vi "LightHouse Refrigerator Tool.vi"() -> ()   [LabVIEW 2021]
uses:
  Common/LabVIEW GEA2 Toolkit/GEA3/type defs/Data In.ctl
  Common/LabVIEW GEA2 Toolkit/GEA3/type defs/Source_Destination.ctl
  Common/LabVIEW GEA2 Toolkit/GEA3/type defs/ERD Write Data In.ctl
  Common/LabVIEW GEA2 Toolkit/GEA3/type defs/Data Type.ctl
  Common/LabVIEW GEA2 Toolkit/GEA3/type defs/ERD Read Data Out.ctl
  Common/LabVIEW GEA2 Toolkit/GEA3/type defs/ERD Read Data In.ctl
  Dryer Tool (Commercial 2)/JL Dryer Tool Support/type defs/Programming.ctl
  Dryer Tool (Commercial 2)/JL Dryer Tool Support/type defs/Flash_Results.ctl
  Dryer Tool (Commercial 2)/JL Dryer Tool Support/type defs/Select _Graph_JL.ctl
  Common/GEA2 Script/typedefs/Script Info.ctl
  Dryer Tool (Commercial 2)/JL Dryer Tool Support/UTL_JL Scaling Factor Folder/Controls/ENUM_JL Scaling Factor_.ctl
  <vilib>/Platform/fileVersionInfo.llb/FileVersionInformation.ctl
  Dryer Tool (Commercial 2)/JL Dryer Tool Support/type defs/Choose_ERD_List.ctl
  Common/Diagnostics Decode/Type Defs/Diag_FaultTableStatus.ctl
  Common/Diagnostics Decode/Type Defs/Diag_FaultTableEntry.ctl
  Common/Diagnostics Decode/Type Defs/Diag_EntityManifestType.ctl
  Common/Diagnostics Decode/Type Defs/Diag_FaultSeqEntry.ctl
  Automation2/Product Specific/Clothes Care/Justice League/Product Testcode/Diagnostics/TypeDefs/Centauro Diagnostic V3 SnapShot.ctl
  Dryer Tool (Commercial 2)/JL Dryer Tool Support/type defs/JL_Diagnost V3 Cycle History.ctl
  Dryer Tool (Commercial 2)/JL Dryer Tool Support/type defs/ERD_Graph.ctl
  Dryer Tool (Commercial 2)/JL Dryer Tool Support/type defs/ERDList.ctl
  Dryer Tool (Commercial 2)/JL Dryer Tool Support/type defs/ERD_Loop_States_JL.ctl
  Dryer Tool (Commercial 2)/JL Dryer Tool Support/type defs/Version.ctl
  Dryer Tool (Commercial 2)/JL Dryer Tool Support/type defs/BootloaderVersion.ctl
  Common/LabVIEW GEA2 Toolkit/GEA3/type defs/Data Out.ctl
  D:/Common/LabVIEW GEA2 Toolkit/source/GEA3 DLL Source/GeaCommunication.dll
  Common/LabVIEW GEA2 Toolkit/source/GEA3 DLL Source/GeaCommunication.dll
  Common/GExplorer Support/typedefs/GExplorer_Data_Cluster.ctl
  Dryer Tool (Commercial 2)/JL Dryer Tool Support/type defs/ERD_Data_Loop_Control.ctl
  Dryer Tool (Commercial 2)/JL Dryer Tool Support/type defs/Error_Command.ctl
  Dryer Tool (Commercial 2)/JL Dryer Tool Support/type defs/DAQ_States.ctl
  Dryer Tool (Commercial 2)/JL Dryer Tool Support/type defs/Cont_Send_States.ctl
  Refrigerator Tool Support/Controls/All_Bundled_Data_RT.ctl
  Dryer Tool (Commercial 2)/JL Dryer Tool Support/type defs/ERD_Always_Show_JL.ctl
  Dryer Tool (Commercial 2)/JL Dryer Tool Support/type defs/CSV_File_String_Arrays.ctl
  Dryer Tool (Commercial 2)/JL Dryer Tool Support/type defs/Fault Table Array.ctl
  Dryer Tool (Commercial 2)/JL Dryer Tool Support/type defs/Fault_Table_Info.ctl
  Dryer Tool (Commercial 2)/JL Dryer Tool Support/type defs/DAQ_Control_Command.ctl
  Dryer Tool (Commercial 2)/JL Dryer Tool Support/type defs/ERD_Loop_Control_Command.ctl
  Dryer Tool (Commercial 2)/JL Dryer Tool Support/type defs/GEA2_Control_Command.ctl
  <vilib>/DAQmx/read.llb/DAQmx Read (Digital 1D Bool NChan 1Samp 1Line).vi
  <vilib>/DAQmx/write.llb/DAQmx Write (Analog 1D DBL NChan 1Samp).vi
  <vilib>/DAQmx/write.llb/DAQmx Write (Digital 1D Bool NChan 1Samp 1Line).vi
  Common/LabVIEW GEA2 Toolkit/GEA3/advanced/GEA2 Message Received Event Handler.vi
  <vilib>/DAQmx/create/channels.llb/DAQmx Create Channel (DI-Digital Input).vi
  <vilib>/DAQmx/create/channels.llb/DAQmx Create Channel (AO-Voltage-Basic).vi
  <vilib>/DAQmx/create/channels.llb/DAQmx Create Channel (DO-Digital Output).vi
  <vilib>/DAQmx/miscellaneous.llb/DAQmx Fill In Error Info.vi
  Common/LabVIEW GEA2 Toolkit/GEA3/library/GEA2_Toolkit.lvlib
panel:
  in  "Board Index":u8=1 min=1 max=10 step=1
  in  "Pause(mls)":u32=100
  out "Rate":u32=100
  out "State":T1=enum."Read ERDs"
  in  "Data ON":bool=TRUE
  in  "Stop":bool
  in  "UI Launch":bool
  in  "Tab Control":T2(tab)=enum."ERD List"
  out "CSV File Log Path":path=path "D:/QA/Commercial 2/Dryer_Xolo/ProbandoC2_24-11-21_15-05-37.csv"
  out "Version":T3
  in  "Read ERD List":T4[](array[typedef])=[{"ERD Number"=49, "Data Type"=enum."string"}] {"ERD Number" format="%.0x"}
  in  "Read ERD":bool
  in  "Write ERD List":T5[](array[typedef])=[{"ERD Number"=49, "Data Type"=enum."string", "Data"="01"}] {"ERD Number" format="%.0x"}
  in  "Write ERD":bool
  out "Read ERD Data Out":T7[](array[typedef])=[{"ERD Number"=49, "Data"="00 00 00 16"}] {"ERD Number" format="%.0x"}
  out "Boot Loader Version":T8
  in  "GEA Inputs":T9={"Source"=229, "Destination"=2} {"Destination" format="%.0x"; "Source" format="%.0x"}
  in  "Exit Botloader":bool
  in  "Enum":enum16{"All", "MC", "UI"}(ring)
  in  "Entry Botloader":bool
  out "FileVersionInfo":T10
  out "LabView/Version Number":string
  in  "Tool Version":bool=TRUE
  out "GEA2 Log":string
  in  "Save Log":bool
  in  "GEA2 Log Length":i32=100000
  in  "Clear":bool
  in  "Ignore this CMD":string
  in  "Filter Data":bool=TRUE
  in  "Programming":T11={"Program"=FALSE, "File Path"=path "", "Program Ind"=FALSE, "Reset Board"=FALSE, "Enter Bootloader"=FALSE, "Result"=9} {"Result" items=["ImageRejected", "BoardNotFound", "UnableToGetGeaConfiguration", "WriteToFlashNotAllowed", "ImageDownloadedSuccessfully", "ImagePresent", "WriteToFlashFailed", "EraseFailed", "CrcFailed", ""]}
  in  "Flash Latest":bool
  in  "Send Button":bool
  in  "GEA2 Send":T13={"Source"=228, "Destination"=2, "Command"=0, "Message"=""} {"Command" format="%02x"; "Destination" format="%02x"; "Source" format="%02x"}
  in  "Msg Rate (ms)":u32=1000 min=50 step=50
  in  "Start Send":bool
  out "Converted Data Out":T14 {"CRC" format="%04x"; "Length" format="%02x"; "Command" format="%02x"; "Destination" format="%02x"; "Source" format="%02x"}
  in  "ERD Graph Cntrl":cluster{"ERD 3":T15, "ERD 2":T15, "ERD 1":T15}={"ERD 3"={"ERD #"=62250, "Data Type"=enum."uint32_t", "Scaler"=1024}, "ERD 2"={"ERD #"=62250, "Data Type"=enum."uint32_t", "Scaler"=1024}, "ERD 1"={"ERD #"=62250, "Data Type"=enum."uint32_t", "Scaler"=1024}} {"ERD 1"."Scaler" min=1; "ERD 1"."ERD #" format="%.0x"; "ERD 2"."Scaler" min=1; "ERD 2"."ERD #" format="%.0x"; "ERD 3"."Scaler" min=1; "ERD 3"."ERD #" format="%.0x"}
  in  "ERD Graphing ON":bool
  out "ERD Graph  Ind":T16
  in  "Graphing ON":bool
  in  "Select Graph":T17
  out "Outlet Thermistor":u16(graph)
  out "Filtered Moisture":u16(graph)=768
  out "Raw Moisture":u16(graph)=155
  out "All Loads":u16[][](graph)=[[0, 0, 0, 768, 100, 200, 300, 400, 575, 600, 700]]
  out "ERD 1":dbl(graph)
  out "ERD 2":dbl(graph)
  out "Inlet Thermistor":u16(graph)
  out "ERD 3":dbl(graph)
  in  "Get Faults":bool
  in  "Clear Fault Table Buffer":bool
  in  "Clear Fault Seq Buffer":bool
  out "Fault Sequence Entries":T18[](array[typedef])
  out "Fault Seq Status":T19
  out "Fault Table Entries":T20[](array[typedef])
  out "Fault Table Status":T19
  out "Diagnostic Entity Manifest":T21
  out "Major Version":u8
  out "Minor Version":u8
  out "Fault Set?":bool
  in  "Filter by Count":bool=TRUE
  out "Centauro Fault Snapshot":T22
  in  "LED Control":T23
  in  "Normal Temp V":bool=TRUE
  in  "Manual Inlet":dbl format="%#_13g"
  in  "Manual Outlet":dbl format="%#_13g"
  in  "Init/Scale":T24=enum."Scale Voltage"
  in  "Scalling":T25={"Low  "=1531.0, " High"=6859.0, "Actual Low"=1.0, "Actual High"=4.9}
  in  "Desired FilteredMoisture":dbl=2400.0 min=1000.0 max=6300.0 step=5.0
  out "Drum":bool
  out "Centrifugal Switch":bool caption="Cent SW"
  out "Drum Direction":string
  in  "CentSWControl":bool
  in  "CentSWControlType":bool=TRUE
  out "Steam":bool
  out "Drum Light":bool
  out "Outer Coil":bool
  out "Inner/Gas Coil":bool
  in  "Dither (V)":dbl=0.05 min=0.0 max=1.0 step=0.001 format="%_3g"
  in  "Outlet Therm (F)":dbl(knob)=75.0 min=49.0 max=201.0 step=1.0 scale=50.0..200.0
  in  "Inlet Therm (F)":u16(knob)=75 min=49 max=501 step=1 scale=50.0..500.0
  in  "Moisture (V)":dbl(slide)=1.8451000000000002 min=0.0 max=5.0 step=0.0001 scale=0.0..5.0 scale format="%#.2f"
  in  "AC Power":bool=TRUE
  in  "Door Status":bool=TRUE
  in  "Start Signal":bool
  out "DAQ Status":string="Exit"
  in  "Turn On DAQ":bool
  out "DAQ On?":bool
  out "Inlet Voltage":dbl
  out "Outlet Voltage":dbl
  in  "Model":enum16{"Estar Centauro", "GFL"}(ring)
  in  "Get Cycle Data":bool
  in  "Filter by Status Count":bool=TRUE
  out "JL Cycle History":T26
  out "output cluster":T19
  out "Bits":i32
  in  "Script Log Path":path
  in  "Run Script":bool
  out "Script Pass/Fail?":bool
  out "Script Report Text":string
  in  "stop script":bool
  in  "Script Path":path
  out "Script Info":T27 {"Overall Script File Progress" scale=0.0..1.0; "Elapsed time (s)" format="%#.1f"; "Current Script Progress" scale=0.0..1.0}
  out "Script Error Out":errorcluster
  in  "Load ERD List":T28
  in  "ERD Default List":T29=[{"Boolean"=TRUE, "ERD Number"=1792, "ERD Nanme"="Erd_ResetCount", "Data_Type"=enum."string"}] {"ERD Number" format="%x"}
  in  "ERD's List Ticket Testing":T29 {"ERD Number" format="%x"}
  in  "Wifi State":T30(ring)
  in  "Set Wifi State(ERD 6003)":bool
  in  "Turn on Wifi":bool
  in  "Turn off Wifi":bool
  out "Wifi Network State":string
  out "Wifi Password":string
  out "Wifi Network Name":string
  out "Mac Address":string
  in  "Get Wifi Data":bool
  out "Error Out":errorcluster
  in  "Error In":errorcluster
  # "Ver. 0.1"
  # "ERD_Graph_All.ctlERD_Graph_All.ctlMust input av valid ERD# and Data Type DO NOT Leave Blank If no scaler use value of 01"
  # "Filtered Moisture"
  # "Voltage (DAQ)"
  # "Measured Range"
  # "Centrifugal Switch"
  # "On"
  # "Normal"
  # "Off"
  # "Manual"
  # "Wifi State is Writing to ERD 6003 and communicating with the wifi board directly.  It will remain in the state you wrote it to until another command is recieved. \n\nOnly Write to invalid if you are testing the board in Invalid state."
  # "After turning on Wifi , wait about 30 seconds and press the Get Wifi Data button.  Network state should be 1, apmode.\n\nAll this is doing is Writing the ERD 0xF115 Service Request to request connect, or disconnect."
  # "Contact:\n\nTerrance Bradford\nTerrance.Bradford@geappliances.com"
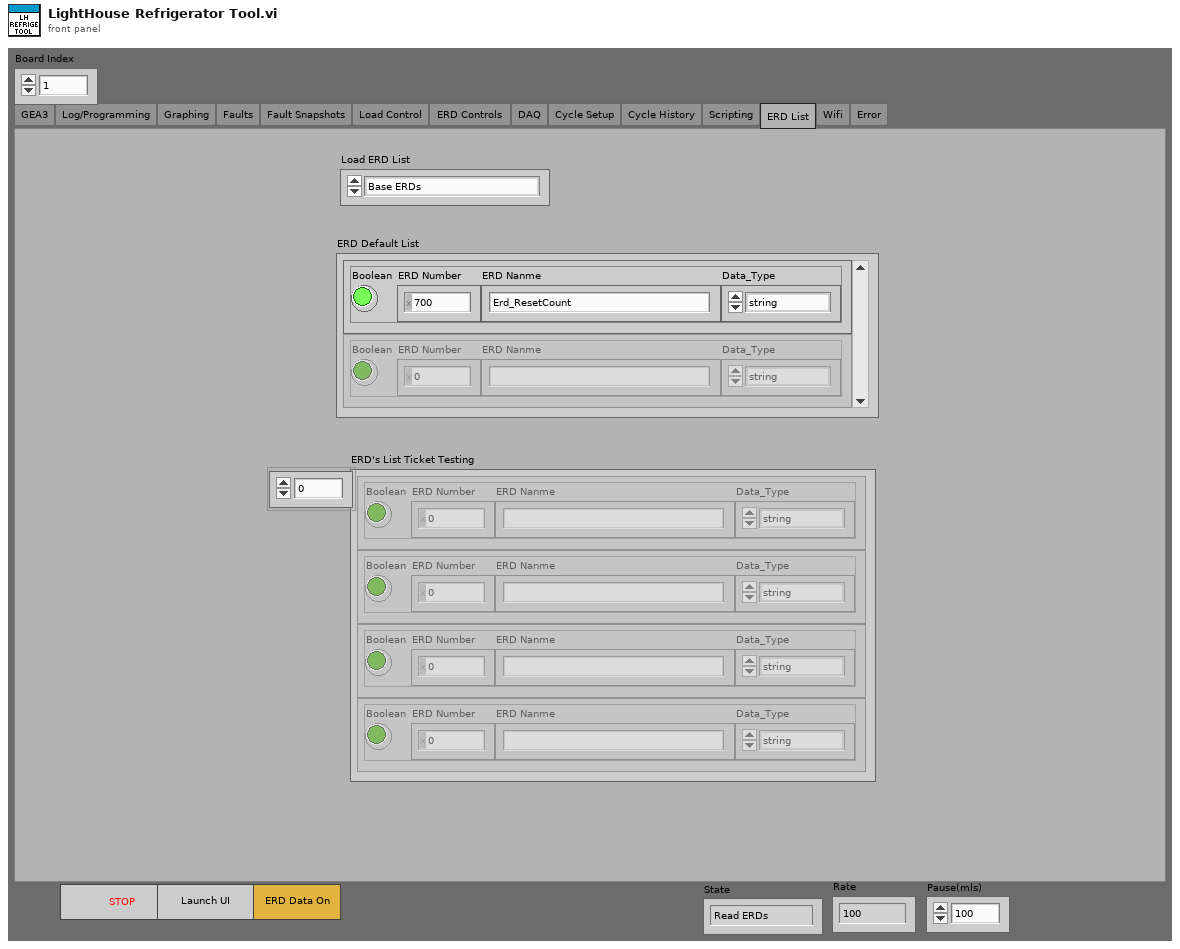
[diagram p1: front panel]
types:
  T1 = typedef "ERD_Loop_States_JL.ctl" = enum16{"Init", "Build ERD Read List", "Read ERDs", "Get Version", "Check Load Size", "Update UI", "Update Graphs", "Read Faults", "Log Data", "Pause", "Shutdown"}
  T2 = enum32{"GEA3", "Log/Programming", "Graphing", "Faults", "Fault Snapshots", "Load Control", "ERD Controls ", "DAQ", "Cycle Setup", "Cycle History", "Scripting", "ERD List", "Wifi", "Error"}
  T3 = typedef "Version.ctl" = cluster{"Build Number":string, "Build Hash ":string, "Application Version":string, "Parametric Version":string, "UI App Version":string}
  T4 = typedef "ERD Read Data In.ctl" = cluster{"ERD Number":u16, "Data Type":enum16{"string", "boolean", "uint8_t", "uint16_t", "uint32_t", "uint64_t", "int8_t", "int16_t", "int32_t", "int64_t"}}
  T5 = typedef "ERD Write Data In.ctl" = cluster{"ERD Number":u16, "Data Type":T6, "Data":string}
  T6 = typedef "Data Type.ctl" = enum16{"string", "boolean", "uint8_t", "uint16_t", "uint32_t", "uint64_t", "int8_t", "int16_t", "int32_t", "int64_t"}
  T7 = typedef "ERD Read Data Out.ctl" = cluster{"ERD Number":u16, "Data":string}
  T8 = typedef "BootloaderVersion.ctl" = cluster{"UI BL Version":string, "MC BL Version":string}
  T9 = typedef "Source_Destination.ctl" = cluster{"Source":u8, "Destination":u8}
  T10 = typedef "FileVersionInformation.ctl" = cluster{"FileVersion":string, "ProductName":string, "InternalName":string, "CompanyName":string, "LegalCopyright":string, "FileDescription":string}
  T11 = typedef "Programming.ctl" = cluster{"Program":bool, "File Path":path, "Program Ind":bool, "Reset Board":bool, "Enter Bootloader":bool, "Result":T12}
  T12 = typedef "Flash_Results.ctl" = i32
  T13 = typedef "Data In.ctl" = cluster{"Source":u8, "Destination":u8, "Command":u8, "Message":string}
  T14 = typedef "Data Out.ctl" = cluster{"Source":u8, "Destination":u8, "Command":u8, "Length":u8, "CRC":u16, "Message":string}
  T15 = typedef "ERD_Graph.ctl" = cluster{"ERD #":u16, "Data Type":T6, "Scaler":u32}
  T16 = cluster{"ERD Value 1":dbl, "ERD Value 2":dbl, "ERD Value 3":dbl}
  T17 = typedef "Select _Graph_JL.ctl" = enum16{"All Loads", "Inlet Thermistor", "Outlet Thermistor", "Raw Moisture", "Filtered Moisture", "ERD 1", "ERD 2", "ERD 3"}
  T18 = typedef "Diag_FaultSeqEntry.ctl" = cluster{"Cycle #":u32, "Time":u32, "F Code":string, "F Active":bool}
  T19 = typedef "Diag_FaultTableStatus.ctl" = cluster{"Cur Index":u16, "Count":u16, "Ov Cnt":u16}
  T20 = typedef "Diag_FaultTableEntry.ctl" = cluster{"Cycle #":u32, "Time":u32, "F Code":string, "F Count":u16, "F Active":bool}
  T21 = typedef "Diag_EntityManifestType.ctl" = cluster{"ID":u8, "Data Ver Maj":u8, "Data Ver Min":u8, "Fault Table?":bool, "Fault Table Snap?":bool, "Fault Seq?":bool, "Fault Seq Snap?":bool, "Cycle History Seq?":bool, "Fault Table Entry Count":u16, "Fault Seq Entry Count":u16, "Cycle History Entry Count":u16, "Cycle Count":u32, "Entity Run Time (Min)":u32}
  T22 = typedef "Centauro Diagnostic V3 SnapShot.ctl" = string[][]
  T23 = cluster{"ALL LEDs ON":bool, "ALL LEDs OFF":bool, "Reset LEDs":bool}
  T24 = typedef "ENUM_JL Scaling Factor_.ctl" = enum16{"Init", "Scale Voltage", "Flush Slope"}
  T25 = cluster{"Low  ":dbl, " High":dbl, "Actual Low":dbl, "Actual High":dbl}
  T26 = typedef "JL_Diagnost V3 Cycle History.ctl" = string[][]
  T27 = typedef "Script Info.ctl" = cluster{"Overall Script File Progress":dbl, "Current Script Progress":dbl, "Script":string, "Test":string, "Elapsed time (s)":dbl, "Done?":bool}
  T28 = typedef "Choose_ERD_List.ctl" = enum16{"Base ERDs", "QA ERDs", "MABE ERD List", "EcoDry Evaluation ERD List", "ClothDampnessCheck ERD List"}
  T29 = typedef "ERDList.ctl" = cluster{"Boolean":bool, "ERD Number":u16, "ERD Nanme":string, "Data_Type":enum16{"string", "boolean", "uint8_t", "uint16_t", "uint32_t", "uint64_t", "int8_t", "int16_t", "int32_t", "int64_t"}}[]
  T30 = enum16{"0 - OFF", "1 - App Mode", "2 - Connecting", "3 - Connected", "4 - Connected Off", "5 - Scanning", "6 - Reconnecting", "255 - Invalid"}
  T31 = typedef "All_Bundled_Data_RT.ctl" = cluster{"Version":T3, "ERD_Always Show":T32, "Personality Set":u8, "CSV File String Arrays":T33, "Fault Table Array ":T34, "Boot Loader Version":T8}
  T32 = typedef "ERD_Always_Show_JL.ctl" = cluster{"Inlet Thermistor":u16, "Machine State":string, "Filtered Moisture":u16, "Cycle Selected":string, "HTR 1 / Inner / Top":bool, "HTR 2 / Outer / Bot":bool, "Door Switch":bool, "Drum Light":bool, "Cycle Engine State":string, "Centrifugal Switch":bool, "Drum Motor":bool, "Cycle Count":u32, "Ext. Tumble":bool, "eDry":bool, "Temp Level":string, "Dryness Level":string, "Time Level":string, "Delay Time (min)":u16, "Steam Refresh":bool, "Damp Alert":bool, "Sub-Cycle":string, "Outlet Thermistor":u16, "Target Moisture":u16, "Remaining Cycle Time":u32, "Raw Moisture":u16, "Cycle Name":string, "My Cycle":bool, "Delay Dry":bool, "Detangle":bool, "Control Lock":bool, "Steam Valve":bool, "Door Latch":bool, "Signal Volume":string, "Tune ID":string, "Restr Detect Status":string, "Vent Restriction":string, "Load Size by Contact":string, "Load Size by Temp":string, "EOC Reason":string, "Sensor Dry Status":string, "Dampness State":string, "Target Voltage Reached":bool, "TrimInhibitR1":bool, "TrimInhibitR2":bool, "TrimBothCoilInhibit":bool, "NormalHeatControl":bool, "HeatControl Request":bool, "Cool Down Status":string, "EcoDryInhibitRelay1":bool, "EcoDryInhibitRelay2":bool, "ReverseDrumInhibitRelay1":bool, "ReverseDrumInhibitRelay2":bool, "OverTempHeaterInhibitRequest":bool, "FallbackHeatControlMethodStatus":bool, "IHC TimeSeconds":u32, "ECT TimeSeconds ":u32, "SC Total Drying Time(S')":u32, "TTR Target Voltage (S')":u32, "TCT Drying Time (S's)":u32, "Drum Motor State":enum16{"Off", "Cw", "Ccw", "Max"}, "Load Size by Ag":string, "MaxFIletered Voltage":u16, "Dry Load Detection":string, "Min Sensing Elapse Sec":u32, "Time Multi Sec X100":u32, "Time Adder  Sec":u32, "Temp Multi EcoDry":string, "Temp Multi ExtraLow":string, "Temp Multi Low ":string, "Temp Multi Medium":string, "Temp Multi High":string, "SmoothMoisture":u16, "Eco Dry SEL Status":string, "Eco Dry SEL Result":string, "Eco Dry Cont Status":string, "Eco Dry Relay1 Timer":string, "Eco Dry Relay2 Timer ":string, "Eco Dry Stage 2 Tans ":u32, "WiFiCommissioningPSt":string, "Payment Method":string}
  T33 = typedef "CSV_File_String_Arrays.ctl" = cluster{"ERD Number Array":string[], "ERD Name Array":string[], "ERD Converted String Data":string[]}
  T34 = typedef "Fault Table Array.ctl" = T35[]
  T35 = typedef "Fault_Table_Info.ctl" = cluster{"Cycle Count":u32, " Runtime (min) ":u32, "Fault Status":string, "Fault ID":string, "Fault Count":u16}
  T36 = typedef "Cont_Send_States.ctl" = enum16{"Run", "Shutdown"}
  T37 = typedef "DAQ_States.ctl" = enum16{"Wait for Init", "Rename Devices", "Verify Hardware", "Initialize", "Run", "Shutdown", "Exit"}
  T38 = typedef "ERD_Data_Loop_Control.ctl" = cluster{"Data":variant, "State":T1}
  T39 = typedef "Error_Command.ctl" = enum16{"Initialize", "Handle Errors", "Report Errors"}
  T40 = typedef "GExplorer_Data_Cluster.ctl" = cluster{"Data":variant, "State":enum16{"Add to Log", "Clear", "Shutdown"}}
  T41 = enum8{"Enabled", "Disabled", "Disabled and Grayed Out"}
  T42 = enum16{"UI Application APL", "UI Parametric APL", "MC APL"}
  T43 = typedef "GEA2_Control_Command.ctl" = enum16{"Initialize", "Shutdown"}
  T44 = typedef "ERD_Loop_Control_Command.ctl" = enum16{"Initialize", "Shutdown"}
  T45 = typedef "DAQ_Control_Command.ctl" = enum16{"Initialize", "Shutdown", "Exit"}
  T46 = enum32{"invalid app kind", "Development System", "Run Time System", "Student Edition", "Embedded LabVIEW", "Evaluation", "Custom"}
  T47 = typedef "eventsource.ctl" = u32
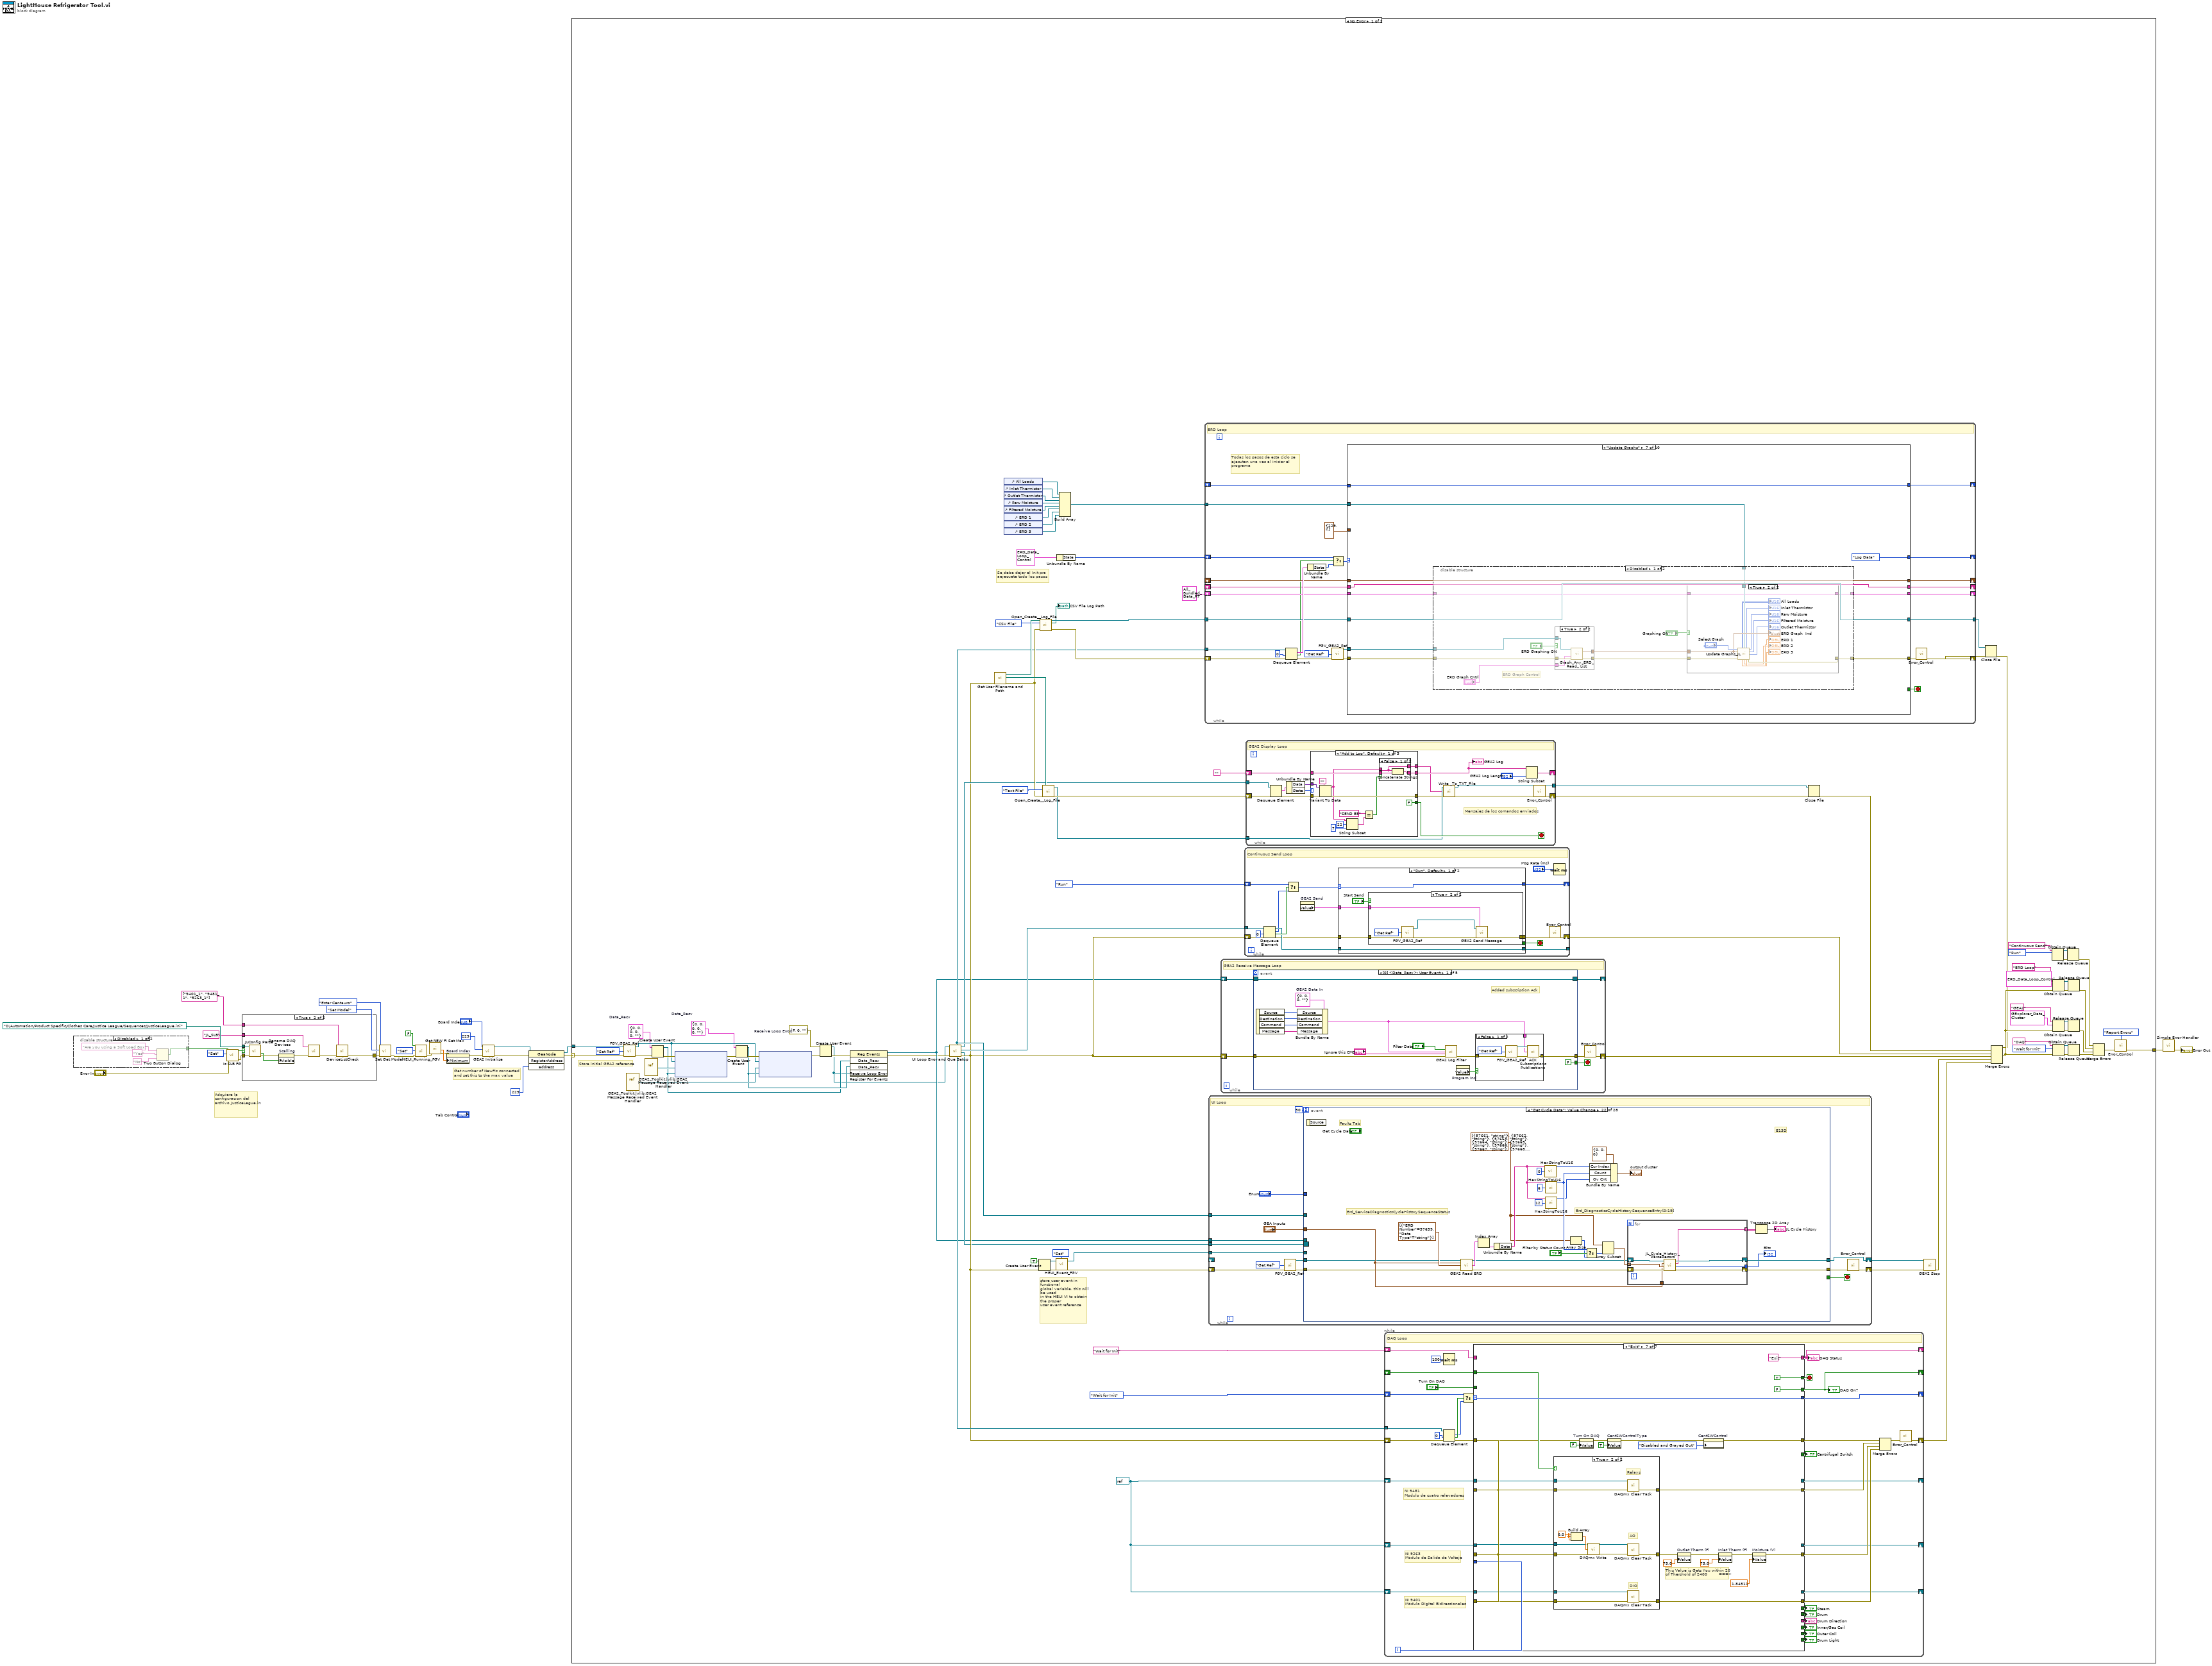
[diagram p0: block diagram]
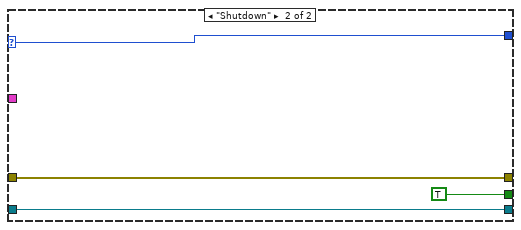
[diagram p5: hidden frame]
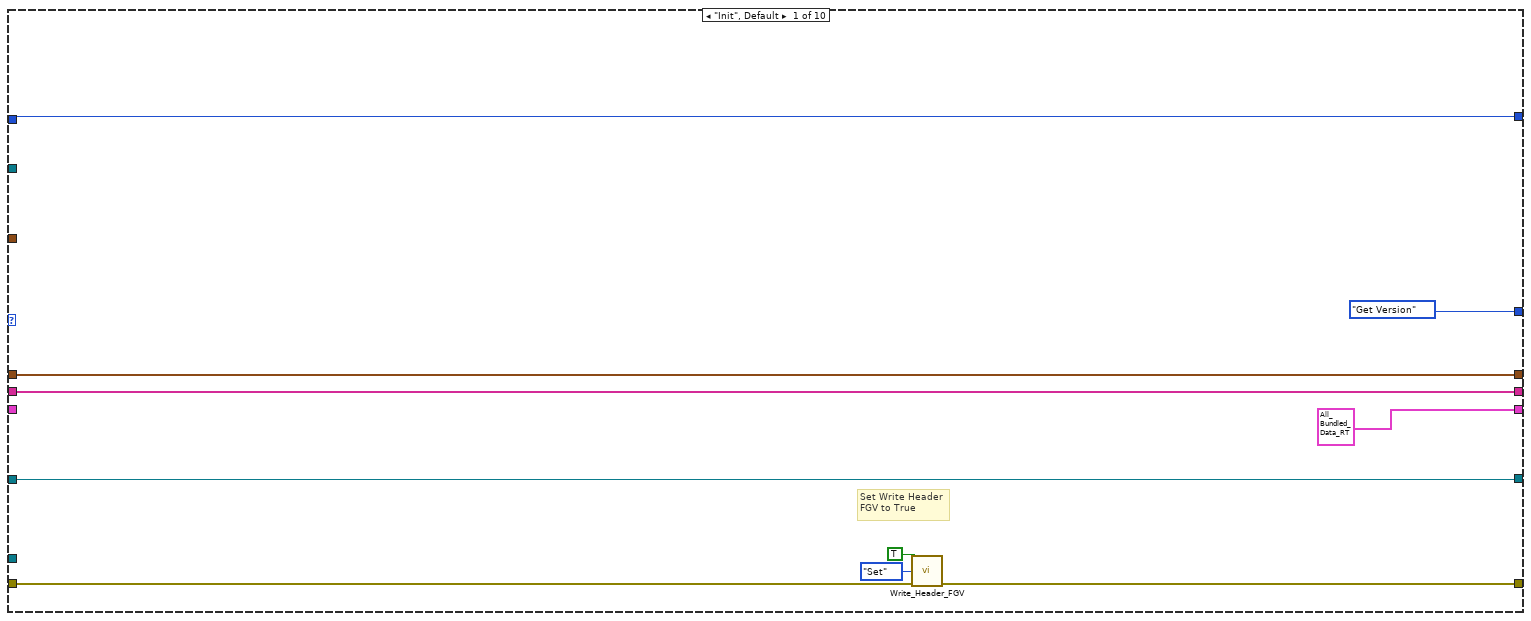
[diagram p6: hidden frame]
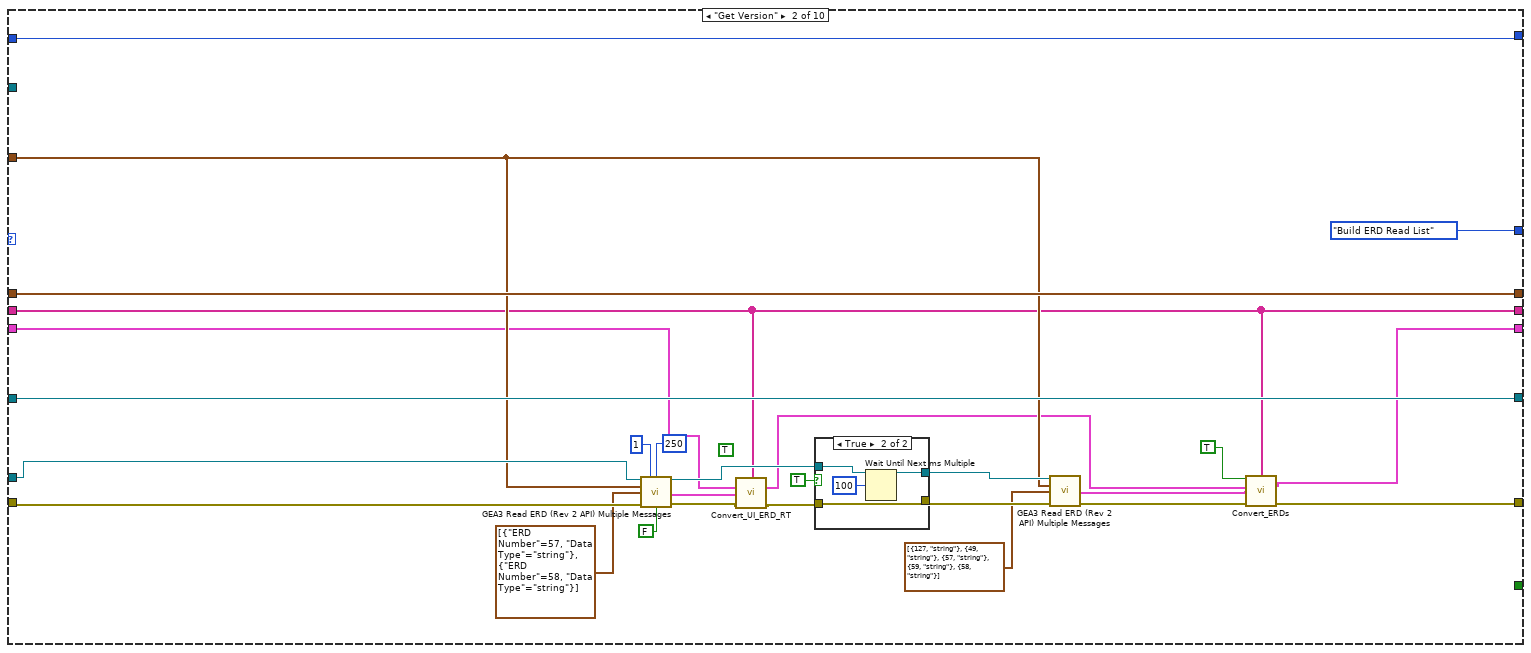
[diagram p7: hidden frame]
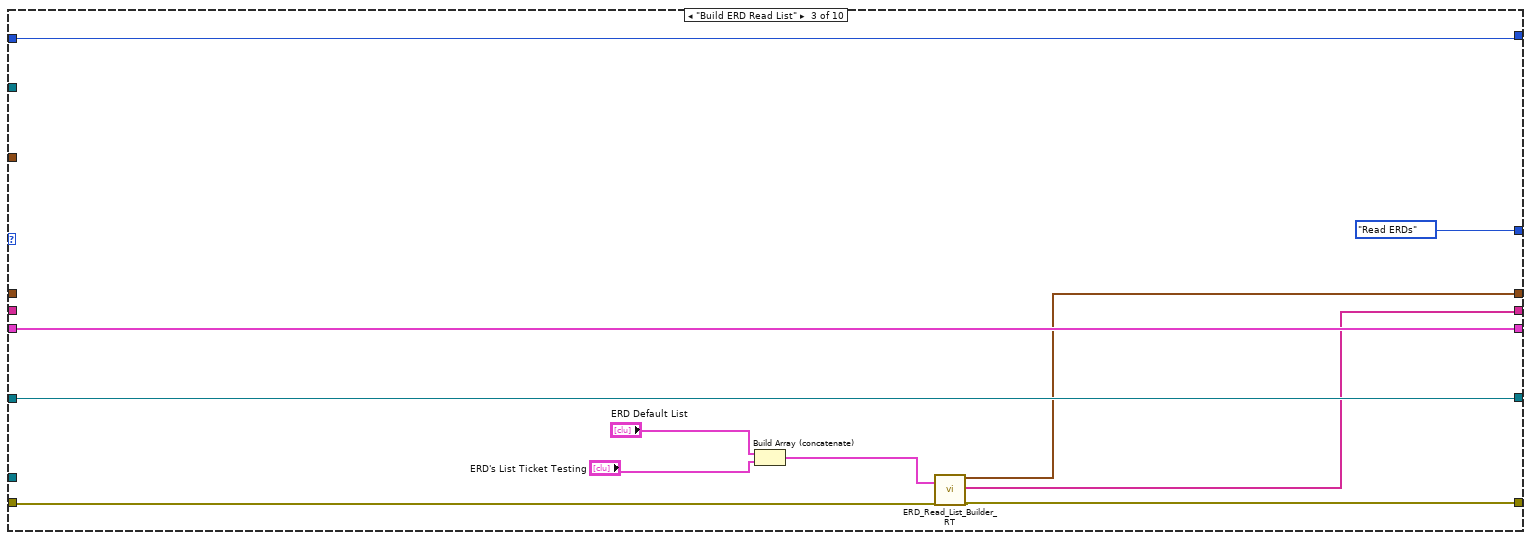
[diagram p9: hidden frame]
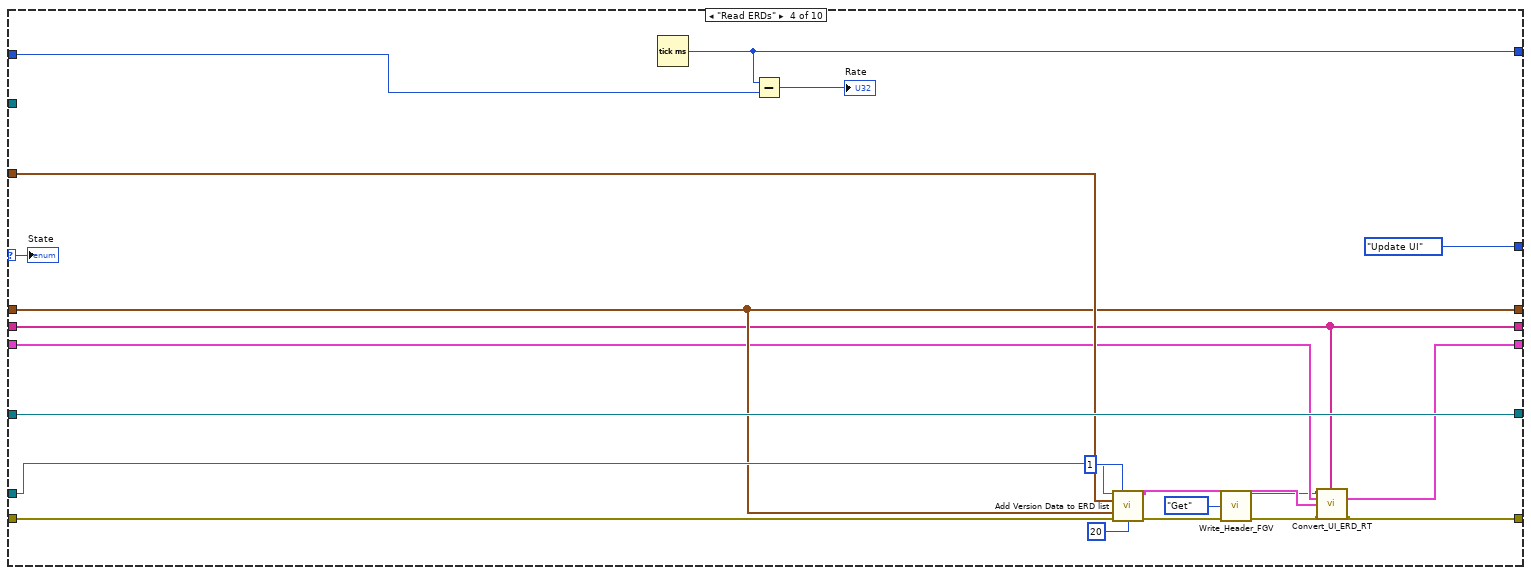
[diagram p10: hidden frame]
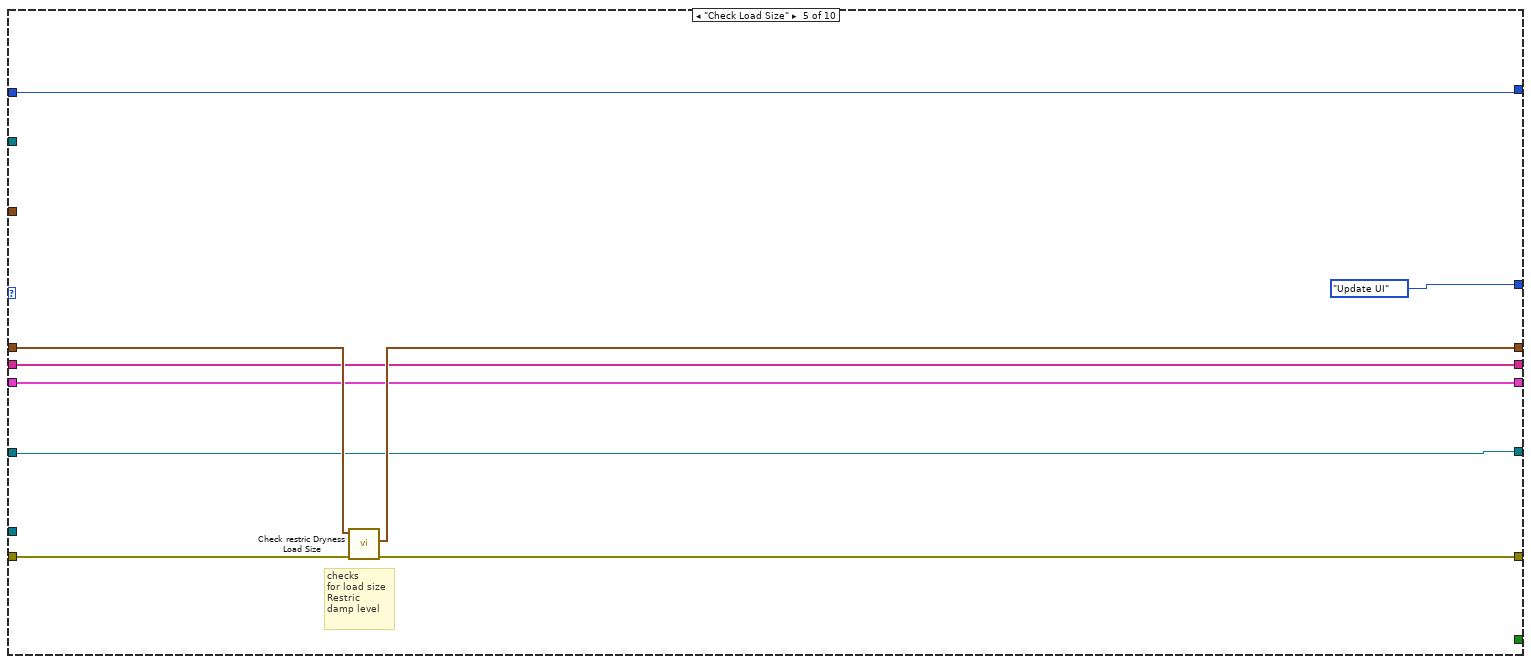
[diagram p11: hidden frame]
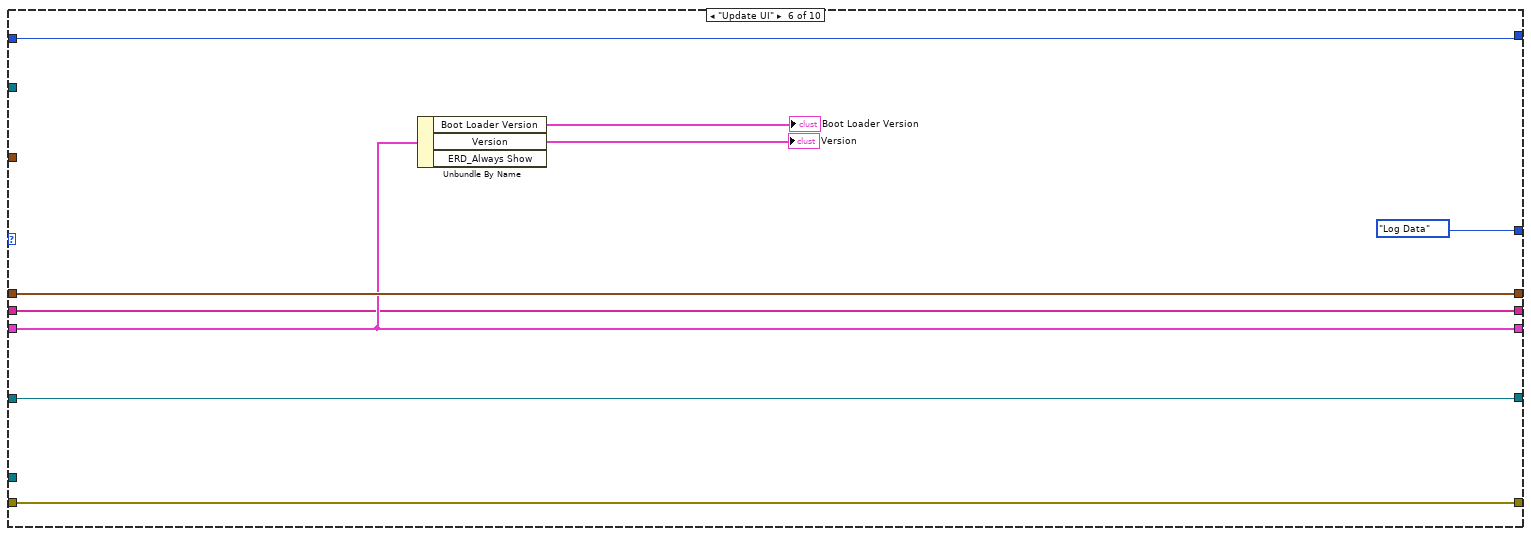
[diagram p12: hidden frame]
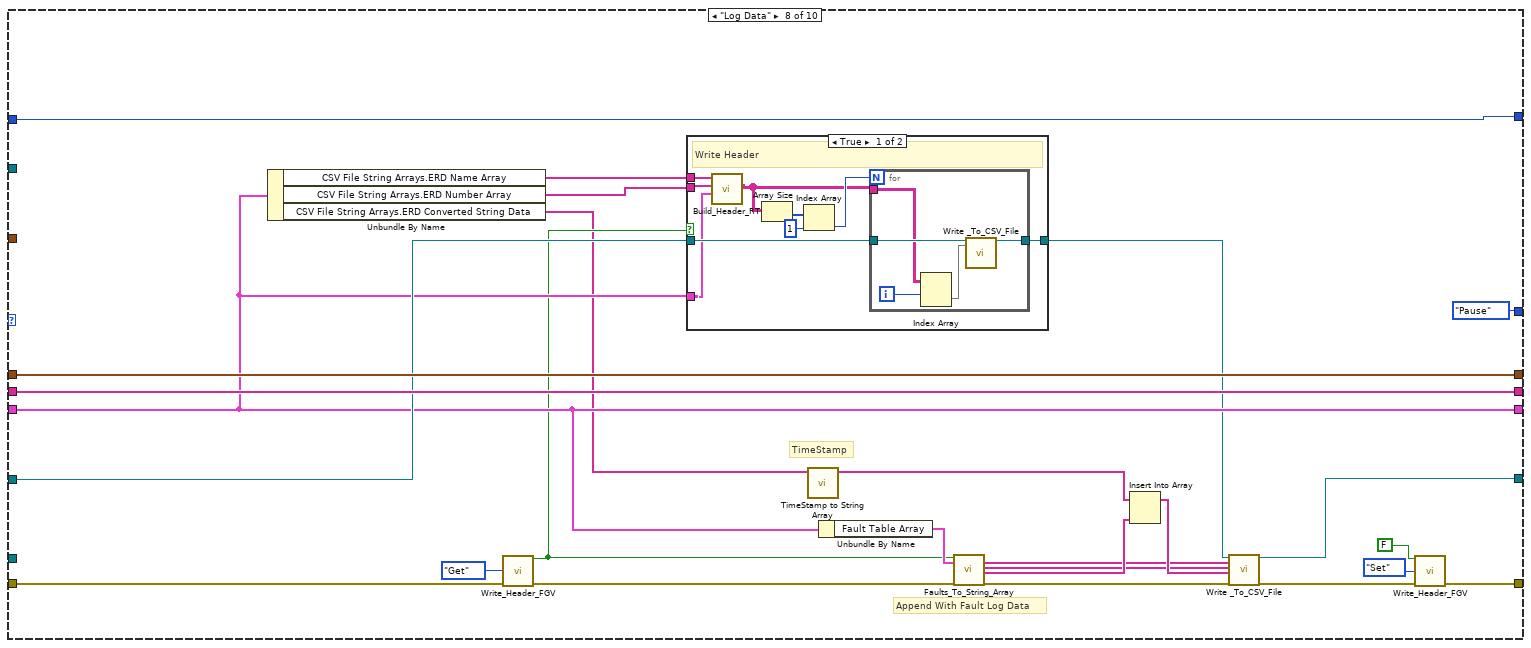
[diagram p16: hidden frame]
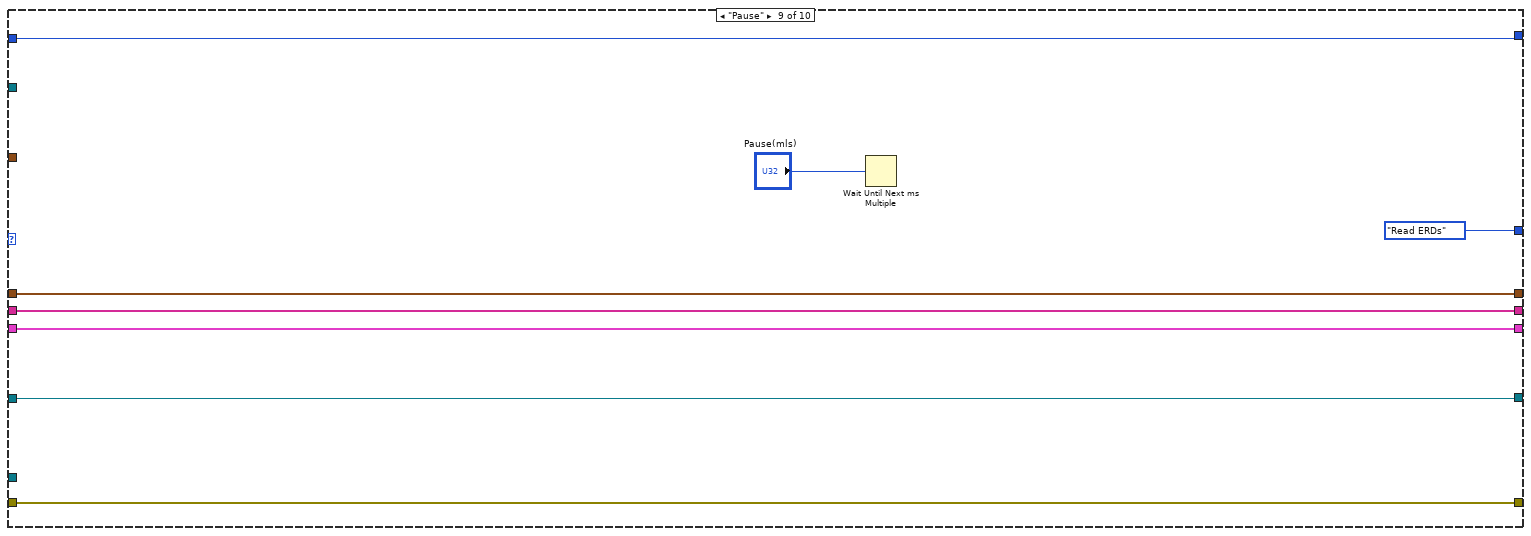
[diagram p18: hidden frame]
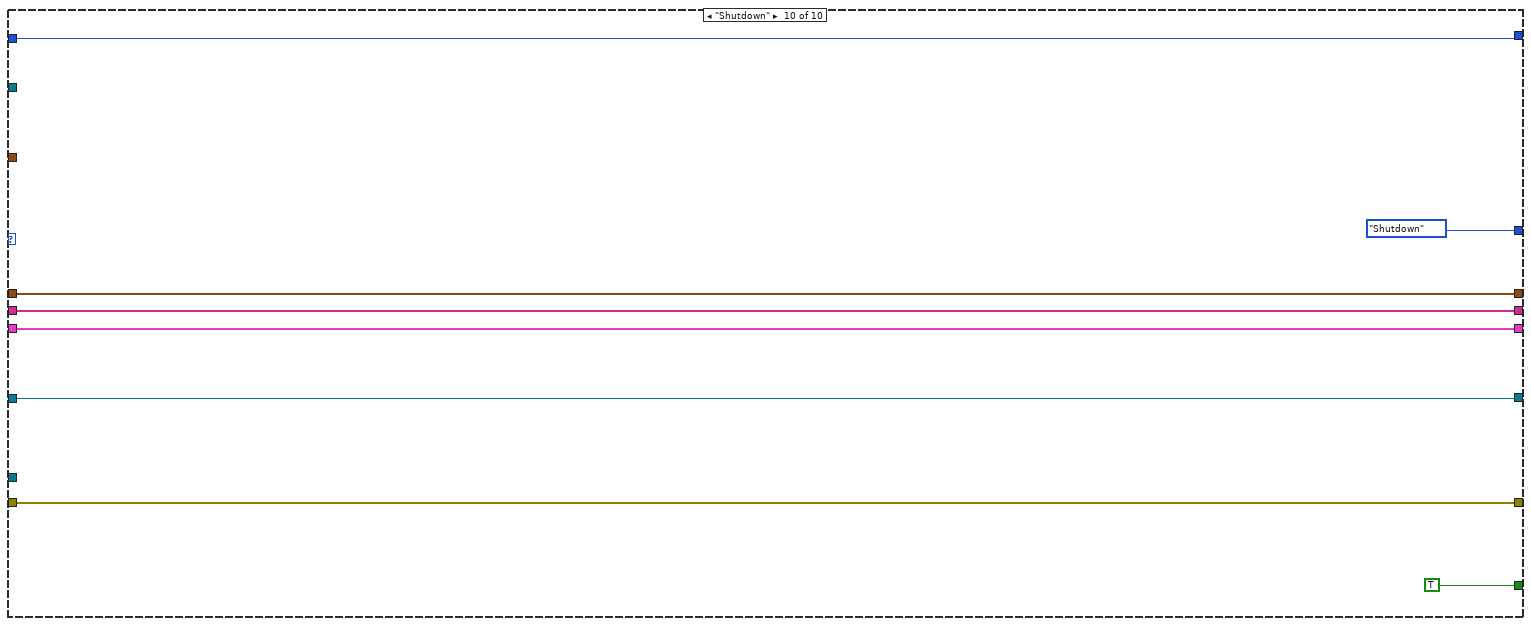
[diagram p19: hidden frame]
diagram:
  # "Adquiere la configuracion del archivo JusticeLegue.in"
  # "Get number of NewFIs connected\nand set this to the max value"
  n1 = disable-structure shown="Disabled" {
    disable-tunnel: [w28 _] -> w16
    frame Disabled {
      n2 = Two Button Dialog(message="Are you using a Soft Load Box?" ("T button name (\"OK\")"), 1:"No" ("F button name (\"Cancel\")"), 2:"Yes" ("message")) -> (T button?=w28:bool)
    }
    frame Enabled {
    }
  }
  n3 = call "Is SLB FG.vi"("Error In"="Error In", "Action"=enum16{"Get", "Set"}."Set", "SLB?"=w16) -> ("Error Out"=w18:errorcluster, "SLB"=w17:bool)  [unwired: 7 in]
  n4 = case shown="True" w17 {
    tunnel: w18 -> [w32 w38]
    tunnel: [w32 w34] -> w13
    tunnel: path "D:/Automation/Product Specific/Clothes Care/Justice League/Sequences/JusticeLeague.ini" ("Config File Path") -> [_ w39]
    tunnel: "JL_SLB" ("cDAQ Name") -> [_ w36]
    tunnel: string[] ["9401_1", "9481_1", "9263_1"] ("Device List") -> [_ w35]
    frame False {
    }
    frame True {
      n5 = call "JLConfig Parse.vi"("Config File Path"=w39, "Error In"=w38) -> ("Calibrate"=w41:bool, "Error Out"=w40:errorcluster)  [unwired: 9 in, 3 out]
      n6 = property on="Scalling" class="Clust (strict)"(error in=w40, "Visible"=w41) -> (error out=w33:errorcluster)  [unwired: 1 in, 1 out]
      n7 = call "Rename DAQ Devices.vi"("cDAQ Name"=w36, "Error In"=w33) -> ("Error Out"=w37:errorcluster)  [unwired: 13 in]
      n8 = call "DeviceListCheck.vi"("Device List"=w35, "Error In"=w37) -> ("Error Out"=w34:errorcluster)  [unwired: 11 in, 2 out]
    }
  }
  n9 = call "Set Get Model.vi"("Error In"=w13, "Action"=enum16{"Set Model", "Get Model"}."Set Model", "Model"=enum16{"Estar Centauro", "GFL"}."Estar Centauro") -> ("Error Out"=w12:errorcluster)  [unwired: 7 in, 1 out]
  n10 = call "HEUI_Running_FGV.vi"("Running?"=FALSE, "Action"=enum16{"Get", "Set"}."Set", "Error In"=w12) -> ("Error Out"=w25:errorcluster)  [unwired: 11 in, 1 out]
  n11 = call "Get NEW FI Set Max.vi"("error in (no error)"=w25) -> ("Error Out"=w8:errorcluster, "Get Max_Out"=w9:dbl)  [unwired: 9 in]
  n12 = property on="Board Index" class="DigNum (strict)"(error in=w8, "Minimum"=w9) -> (error out=w7:errorcluster)  [unwired: 1 in, 1 out]
  n13 = call "GEA2 Initialize.vi"("Board Index"="Board Index", "Source Address"=u8 229, "error in"=w7) -> ("GEA2 Reference Out"=w5:refnum<k24>, "error out"=w2:errorcluster)  [unwired: 10 in, 1 out]
  n14 = invoke class="GeaNode" method="RegisterAddress"(reference=w5, error in=w2, "address"=u8 229 ("Source Address")) -> (reference out=w3:refnum<k24>, error out=w4:errorcluster)  [unwired: 1 in, 2 out]
  n15 = case shown="No Error" w4 {
    selector: w4 -> [w110 w1333]
    tunnel: [w112 w1333] -> w27
    tunnel: w3 -> [w62 _]
    frame No Error {
      w43 = T14 {"Source"=0, "Destination"=0, "Command"=0, "Length"=0, "CRC"=0, "Message"=""}  # Data_Recv
      w45 = T14 {"Source"=0, "Destination"=0, "Command"=0, "Length"=0, "CRC"=0, "Message"=""}  # Data_Recv
      w53 = errorcluster {"status"=FALSE, "code"=0, "source"=""}  # Receive Loop Error
      w67 = refnum<k21> refnum ("task out")
      # "Se debe dejar el Init pra aejecuete todo los pasos"
      # "store user event in functional\nglobal variable, this will be used\nin the HEUI VI to obtain the proper\nuser event reference"
      # "Store initial GEA2 reference"
      n16 = call "FGV_GEA2_Ref.vi"("GEA2 Reference In"=w62, "Action"=enum16{"Set Ref", "Get Ref"}."Set Ref", "Error In"=w110) -> ("GEA2 Reference Out"=w56:refnum<k24>, "Error Out"=w44:errorcluster)  [unwired: 11 in]
      n17 = vi-ref "GEA2_Toolkit.lvlib:GEA2 Message Received Event Handler.vi"() -> (w54:refnum<vi>)
      n18 = vi-ref "GEA2_Toolkit.lvlib:GEA2 Message Received Event Handler.vi"() -> (w55:refnum<vi>)
      n19 = Create User Event(user event datatype=w45, error in=w44) -> (user event=w49:refnum<user-event>, error out=w58:errorcluster)
      n20 = node(w58, w56, w55, w49) -> (w59:errorcluster)  [unwired: 1 in, 1 out]
      n21 = Create User Event(user event datatype=w43, error in=w59) -> (user event=w50:refnum<user-event>, error out=w57:errorcluster)
      n22 = node(w57, w56, w54, w50) -> (w52:errorcluster)  [unwired: 1 in, 1 out]
      n23 = Create User Event(user event datatype=w53, error in=w52) -> (user event=w46:refnum<user-event>, error out=w51:errorcluster)
      n24 = register-events(error in=w51, w49, w50, w46) -> (reference out=w48:refnum<event-registration>, error out=w47:errorcluster)  [unwired: 1 in]
      n25 = call "UI Loop Error and Que Setup.vi"("error in (no error)"=w47, "Receive Loop"=w46) -> ("error out"=w63:errorcluster, "UI Loop Event Registration"=w61:refnum<event-registration>, "Continuous Send Queue"=w83:refnum<queue>, "GEA Display Queue"=w64:refnum<queue>, "Daq Loop queue"=w66:refnum<queue>, "ERD Queue Loop"=w65:refnum<queue>)  [unwired: 4 in]
      n26 = call "Get User Filename and Path.vi"("error in (no error)"=w63) -> ("error out"=w73:errorcluster, "TXT File Path"=w79:path, "CSV File Path"=w81:path)  [unwired: 8 in]
      n27 = control-ref of="All Loads"() -> (w68:refnum<vi>)
      n28 = control-ref of="Inlet Thermistor"() -> (w69:refnum<vi>)
      n29 = control-ref of="Outlet Thermistor"() -> (w70:refnum<vi>)
      n30 = control-ref of="Raw Moisture"() -> (w71:refnum<vi>)
      n31 = control-ref of="Filtered Moisture"() -> (w72:refnum<vi>)
      n32 = control-ref of="ERD 1"() -> (w98:refnum<vi>)
      n33 = control-ref of="ERD 2"() -> (w96:refnum<vi>)
      n34 = control-ref of="ERD 3"() -> (w97:refnum<vi>)
      n35 = Create User Event(user event datatype=TRUE ("Bool"), error in=w63) -> (user event=w105:refnum<user-event>, error out=w106:errorcluster)
      n36 = call "Open_Create__Log_File.vi"("File Path Control"=w81, "Enum"=enum16{"CSV File", "Text File"}."CSV File", "Error In"=w73) -> ("refnum out"=w99:refnum<file>, "File Path"=→"CSV File Log Path":path, "Error Out"=w108:errorcluster)  [unwired: 10 in]
      n37 = call "Open_Create__Log_File.vi"("File Path Control"=w79, "Enum"=enum16{"CSV File", "Text File"}."Text File", "Error In"=w73) -> ("refnum out"=w78:refnum<file>, "Error Out"=w80:errorcluster)  [unwired: 10 in, 1 out]
      n38 = call "HEUI_Event_FGV.vi"("Event In"=w105, "Action"=enum16{"Get", "Set"}."Set", "Error In"=w106) -> ("Event Out"=w102:refnum<user-event>, "Error Out"=w103:errorcluster)  [unwired: 11 in]
      n39 = Unbundle By Name(T38 {"Data"=variant, "State"=enum."Init"} ("Data")) -> ("State"=w100:T1)
      n40 = Build Array(w68, w69, w70, w71, w72, w98, w96, w97) -> (w95:refnum<vi>[])
      n41 = while "Periodic ERD Query Loop" {
        shift-right: [w193] -> w92
        shift-left: w108 -> [w195]
        tunnel: w65 -> [w196]
        shift-right: [w187] -> _
        shift-left: w100 -> [w189]
        shift-right: [w182] -> _
        shift-left: _ -> [w181]
        tunnel: w99 -> [w180]
        tunnel: [w179] -> w90
        shift-right: [w178] -> _
        shift-left: T31 {"Version"={"Build Number"="", "Build Hash "="", "Application Version"="", "Parametric Version"="", "UI App Version"=""}, "ERD_Always Show"={"Inlet Thermistor"=0, "Machine State"="", "Filtered Moisture"=0, "Cycle Selected"="", "HTR 1 / Inner / Top"=FALSE, "HTR 2 / Outer / Bot"=FALSE, "Door Switch"=FALSE, "Drum Light"=FALSE, "Cycle Engine State"="", "Centrifugal Switch"=FALSE, "Drum Motor"=FALSE, "Cycle Count"=0, "Ext. Tumble"=FALSE, "eDry"=FALSE, "Temp Level"="", "Dryness Level"="", "Time Level"="", "Delay Time (min)"=0, "Steam Refresh"=FALSE, "Damp Alert"=FALSE, "Sub-Cycle"="", "Outlet Thermistor"=0, "Target Moisture"=0, "Remaining Cycle Time"=0, "Raw Moisture"=0, "Cycle Name"="", "My Cycle"=FALSE, "Delay Dry"=FALSE, "Detangle"=FALSE, "Control Lock"=FALSE, "Steam Valve"=FALSE, "Door Latch"=FALSE, "Signal Volume"="", "Tune ID"="", "Restr Detect Status"="", "Vent Restriction"="", "Load Size by Contact"="", "Load Size by Temp"="", "EOC Reason"="", "Sensor Dry Status"="", "Dampness State"="", "Target Voltage Reached"=FALSE, "TrimInhibitR1"=FALSE, "TrimInhibitR2"=FALSE, "TrimBothCoilInhibit"=FALSE, "NormalHeatControl"=FALSE, "HeatControl Request"=FALSE, "Cool Down Status"="", "EcoDryInhibitRelay1"=FALSE, "EcoDryInhibitRelay2"=FALSE, "ReverseDrumInhibitRelay1"=FALSE, "ReverseDrumInhibitRelay2"=FALSE, "OverTempHeaterInhibitRequest"=FALSE, "FallbackHeatControlMethodStatus"=FALSE, "IHC TimeSeconds"=0, "ECT TimeSeconds "=0, "SC Total Drying Time(S')"=0, "TTR Target Voltage (S')"=0, "TCT Drying Time (S's)"=0, "Drum Motor State"=enum."Off", "Load Size by Ag"="", "MaxFIletered Voltage"=0, "Dry Load Detection"="", "Min Sensing Elapse Sec"=0, "Time Multi Sec X100"=0, "Time Adder  Sec"=0, "Temp Multi EcoDry"="", "Temp Multi ExtraLow"="", "Temp Multi Low "="", "Temp Multi Medium"="", "Temp Multi High"="", "SmoothMoisture"=0, "Eco Dry SEL Status"="", "Eco Dry SEL Result"="", "Eco Dry Cont Status"="", "Eco Dry Relay1 Timer"="", "Eco Dry Relay2 Timer "="", "Eco Dry Stage 2 Tans "=0, "WiFiCommissioningPSt"="", "Payment Method"=""}, "Personality Set"=0, "CSV File String Arrays"={"ERD Number Array"=[], "ERD Name Array"=[], "ERD Converted String Data"=[]}, "Fault Table Array "=[], "Boot Loader Version"={"UI BL Version"="", "MC BL Version"=""}} ("All_Bundled_Data_Brass") -> [w177]
        tunnel: w95 -> [w176]
        shift-right: [w174] -> _
        shift-left: _ -> [w173]
        shift-right: [w172] -> _
        shift-left: _ -> [w171]
        stop <- w192 stop-if-true
        # "Todas los pasos de esta ciclo se ejecutan una ves al iniciar el programa"
        # "ERD Loop"
        n42 = Dequeue Element(queue=w196, timeout in ms (-1)=0, error in (no error)=w195) -> (element=w184:T38, timed out?=w175:bool, error out=w194:errorcluster)  [unwired: 1 out]
        n43 = Unbundle By Name(w184) -> ("State"=w190:T1)
        n44 = call "FGV_GEA2_Ref.vi"("Action"=enum16{"Set Ref", "Get Ref"}."Get Ref", "Error In"=w194) -> ("GEA2 Reference Out"=w183:refnum<k24>, "Error Out"=w186:errorcluster)  [unwired: 12 in]
        n45 = Select(t=w189, s=w175, f=w190) -> (s? t:f=w188:T1)
        n46 = case shown="\"Update Graphs\"" w188 {
          selector: w188 -> [_ _ _ w268 _ _ _ _ _ _]
          tunnel: w186 -> [w207 w226 w240 w260 w280 w285 w297 w357 w382 w390]
          tunnel: [w201 w217 w241 w252 w278 w285 w296 w356 w382 w390] -> w191
          tunnel: [_ _ _ _ _ _ _ _ _ TRUE] -> w192
          tunnel: T9 {"Source"=229, "Destination"=2} ("ERD Spam GEA Inputs") -> [_ w219 _ w262 _ _ _ _ _ _]
          tunnel: [ERD_Loop_States_JL."Get Version" ("State") ERD_Loop_States_JL."Build ERD Read List" ("State") ERD_Loop_States_JL."Read ERDs" ("State") ERD_Loop_States_JL."Update UI" ("State") ERD_Loop_States_JL."Update UI" ("State") ERD_Loop_States_JL."Log Data" ("State") ERD_Loop_States_JL."Log Data" ("State") ERD_Loop_States_JL."Pause" ("t") ERD_Loop_States_JL."Read ERDs" ("State") ERD_Loop_States_JL."Shutdown" ("State")] -> w187
          tunnel: w183 -> [_ w227 _ w263 _ _ w294 _ _ _]
          tunnel: [w205 w233 w243 w261 w277 w289 w299 w359 w380 w387] -> w182
          tunnel: w181 -> [w205 w233 _ w261 w279 w289 w299 w359 w380 w387]
          tunnel: w180 -> [w204 w232 w249 w270 w276 w286 w298 w353 w379 w386]
          tunnel: [w204 w232 w249 w270 w276 w286 w298 w358 w379 w386] -> w179
          tunnel: [T31 {"Version"={"Build Number"="", "Build Hash "="", "Application Version"="", "Parametric Version"="", "UI App Version"=""}, "ERD_Always Show"={"Inlet Thermistor"=0, "Machine State"="", "Filtered Moisture"=0, "Cycle Selected"="", "HTR 1 / Inner / Top"=FALSE, "HTR 2 / Outer / Bot"=FALSE, "Door Switch"=FALSE, "Drum Light"=FALSE, "Cycle Engine State"="", "Centrifugal Switch"=FALSE, "Drum Motor"=FALSE, "Cycle Count"=0, "Ext. Tumble"=FALSE, "eDry"=FALSE, "Temp Level"="", "Dryness Level"="", "Time Level"="", "Delay Time (min)"=0, "Steam Refresh"=FALSE, "Damp Alert"=FALSE, "Sub-Cycle"="", "Outlet Thermistor"=0, "Target Moisture"=0, "Remaining Cycle Time"=0, "Raw Moisture"=0, "Cycle Name"="", "My Cycle"=FALSE, "Delay Dry"=FALSE, "Detangle"=FALSE, "Control Lock"=FALSE, "Steam Valve"=FALSE, "Door Latch"=FALSE, "Signal Volume"="", "Tune ID"="", "Restr Detect Status"="", "Vent Restriction"="", "Load Size by Contact"="", "Load Size by Temp"="", "EOC Reason"="", "Sensor Dry Status"="", "Dampness State"="", "Target Voltage Reached"=FALSE, "TrimInhibitR1"=FALSE, "TrimInhibitR2"=FALSE, "TrimBothCoilInhibit"=FALSE, "NormalHeatControl"=FALSE, "HeatControl Request"=FALSE, "Cool Down Status"="", "EcoDryInhibitRelay1"=FALSE, "EcoDryInhibitRelay2"=FALSE, "ReverseDrumInhibitRelay1"=FALSE, "ReverseDrumInhibitRelay2"=FALSE, "OverTempHeaterInhibitRequest"=FALSE, "FallbackHeatControlMethodStatus"=FALSE, "IHC TimeSeconds"=0, "ECT TimeSeconds "=0, "SC Total Drying Time(S')"=0, "TTR Target Voltage (S')"=0, "TCT Drying Time (S's)"=0, "Drum Motor State"=enum."Off", "Load Size by Ag"="", "MaxFIletered Voltage"=0, "Dry Load Detection"="", "Min Sensing Elapse Sec"=0, "Time Multi Sec X100"=0, "Time Adder  Sec"=0, "Temp Multi EcoDry"="", "Temp Multi ExtraLow"="", "Temp Multi Low "="", "Temp Multi Medium"="", "Temp Multi High"="", "SmoothMoisture"=0, "Eco Dry SEL Status"="", "Eco Dry SEL Result"="", "Eco Dry Cont Status"="", "Eco Dry Relay1 Timer"="", "Eco Dry Relay2 Timer "="", "Eco Dry Stage 2 Tans "=0, "WiFiCommissioningPSt"="", "Payment Method"=""}, "Personality Set"=0, "CSV File String Arrays"={"ERD Number Array"=[], "ERD Name Array"=[], "ERD Converted String Data"=[]}, "Fault Table Array "=[], "Boot Loader Version"={"UI BL Version"="", "MC BL Version"=""}} ("All_Bundled_Data_Brass") w214 w248 w251 w272 w287 w290 w352 w378 w385] -> w178
          tunnel: w177 -> [_ w211 w248 w255 w272 w287 w293 w352 w378 w385]
          tunnel: w176 -> [_ _ _ _ _ _ w295 _ _ _]
          tunnel: [w200 w210 w242 w253 w274 w284 w292 w355 w377 w384] -> w174
          tunnel: w173 -> [w200 w210 _ w253 w274 w284 w292 w355 w377 w384]
          tunnel: [w199 w231 w247 w267 w273 w283 w291 w354 w376 w383] -> w172
          tunnel: w171 -> [w199 w231 w247 w266 w273 w283 w291 w354 w376 w383]
          frame "Init", Default {
            # "Set Write Header\nFGV to True"
            n47 = call "Write_Header_FGV.vi"("Write Header ? In"=TRUE, "Action"=enum16{"Get", "Set"}."Set", "Error In"=w207) -> ("Error Out"=w201:errorcluster)  [unwired: 11 in, 1 out]
          }
          frame "Get Version" {
            (unwired) TRUE ("New Header?")
            n48 = call "GEA3 Read ERD (Rev 2 API) Multiple Messages.vi"("GEA2 Reference In"=w227, "Retry Count"=1 ("# of Iterations (Should be 2 except JL)"), "Read Timeout (ms)"=u32 250, "GEA Inputs"=w219, "Read ERD List"=T4[] [{"ERD Number"=57, "Data Type"=enum."string"}, {"ERD Number"=58, "Data Type"=enum."string"}] ("Read ERD List MC"), "Error In"=w226, "Verify ERD Response?"=FALSE) -> ("GEA2 Reference Out"=w225:refnum<k24>, "ERD Data Out"=w212:cluster{"ERD Number":u16, "Data":string}[], "Error Out"=w213:errorcluster)  [unwired: 5 in, 1 out]
            n49 = call "Convert_UI_ERD_RT.vi"("ERD Name"=w210, "All_Bundled_Data_Brass"=w211, "Array"=w212, "Error In"=w213) -> ("All_ERD_Data_Bundled_Brass"=w208:T31, "Error Out"=w209:errorcluster)  [unwired: 10 in]
            n50 = case shown="True" TRUE {
              tunnel: [w235 w239] -> w223
              tunnel: w209 -> [w235 w239]
              tunnel: [w236 w238] -> w222
              tunnel: w225 -> [w236 w238]
              frame False {
              }
              frame True {
                n51 = Wait Until Next ms Multiple(millisecond multiple=u32 100) -> ()  [unwired: 1 out]
              }
            }
            n52 = call "GEA3 Read ERD (Rev 2 API) Multiple Messages.vi"("GEA2 Reference In"=w222, "GEA Inputs"=w219, "Read ERD List"=T4[] [{"ERD Number"=127, "Data Type"=enum."string"}, {"ERD Number"=49, "Data Type"=enum."string"}, {"ERD Number"=57, "Data Type"=enum."string"}, {"ERD Number"=59, "Data Type"=enum."string"}, {"ERD Number"=58, "Data Type"=enum."string"}] ("Read ERD List MC"), "Error In"=w223) -> ("ERD Data Out"=w216:cluster{"ERD Number":u16, "Data":string}[], "Error Out"=w218:errorcluster)  [unwired: 8 in, 2 out]
            n53 = call "Convert_ERDs.vi"("New Header?"=TRUE, "ERD Name"=w210, "All_Bundled_Data_Brass"=w208, "Array"=w216, "Error In"=w218) -> ("All_ERD_Data_Bundled_Brass"=w214:T31, "Error Out"=w217:errorcluster)  [unwired: 9 in]
          }
          frame "Build ERD Read List" {
            n54 = Build Array (concatenate)("ERD Default List", "ERD's List Ticket Testing") -> (w244:T29)
            n55 = call "ERD_Read_List_Builder_RT.vi"("ERD Read List ALL"=w244, "Error In"=w240) -> ("Read ERD List"=w243:T4[], "ERD Name"=w242:string[], "Error Out"=w241:errorcluster)  [unwired: 15 in]
          }
          frame "Read ERDs" {
            n56 = Tick Count (ms)() -> (millisecond timer value=w267:u32)
            n57 = Subtract(x=w267, y=w266) -> (x-y=→"Rate":u32)
            n58 = call "Add Version Data to ERD list.vi"(".NET Refnum in"=w263, "# of Iterations (Should be 2 except JL)"=1, "GEA Inputs"=w262, "Read ERD List MC"=w261, "error in (no error)"=w260, "#ERDs per message"=20) -> ("ERD Data Out out"=w256:T7[], "error out"=w259:errorcluster)  [unwired: 8 in]
            n59 = call "Write_Header_FGV.vi"("Action"=enum16{"Get", "Set"}."Get", "Error In"=w259) -> ("Write Header ? Out"=w254:bool, "Error Out"=w257:errorcluster)  [unwired: 12 in]
            n60 = call "Convert_UI_ERD_RT.vi"("New Header?"=w254, "ERD Name"=w253, "All_Bundled_Data_Brass"=w255, "Array"=w256, "Error In"=w257) -> ("All_ERD_Data_Bundled_Brass"=w251:T31, "Error Out"=w252:errorcluster)  [unwired: 9 in]
            "State" <- w268
          }
          frame "Check Load Size" {
            # "checks \nfor load size \nRestric\ndamp level"
            n61 = call "Check restric Dryness Load Size.vi"("Error In"=w280, "Read ERD List"=w279) -> ("Error Out"=w278:errorcluster, "New ERD Data"=w277:T4[])  [unwired: 8 in]
          }
          frame "Update UI" {
            n62 = Unbundle By Name(w287) -> ("Boot Loader Version"=→"Boot Loader Version":T8, "Version"=→"Version":T3)  [unwired: 1 out]
          }
          frame "Update Graphs" {
            n63 = disable-structure shown="Disabled" {
              disable-tunnel: w297 -> [w311 _]
              disable-tunnel: [w309 _] -> w296
              disable-tunnel: w295 -> [w306 _]
              disable-tunnel: w294 -> [w305 _]
              disable-tunnel: w293 -> [w304 _]
              disable-tunnel: [w303 _] -> w290
              frame Disabled {
                # "ERD Graph Control"
                n64 = case shown="True" "ERD Graphing ON" {
                  tunnel: w311 -> [w328 w333]
                  tunnel: [w328 w332] -> w310
                  tunnel: "ERD Graph Cntrl" -> [_ w331]
                  tunnel: [_ w330] -> w307
                  tunnel: w305 -> [_ w329]
                  frame False {
                  }
                  frame True {
                    n65 = call "Graph_Any_ERD_ Read_ List.vi"("GEA2 Reference In"=w329, "ERD Graph Cntrl"=w331, "Error In"=w333) -> ("ERD Graph  Ind"=w330:T16, "Error Out"=w332:errorcluster)  [unwired: 10 in, 1 out]
                  }
                }
                n66 = case shown="True" "Graphing ON" {
                  tunnel: w310 -> [w312 w327]
                  tunnel: [w312 w326] -> w309
                  tunnel: w307 -> [_ w324]
                  tunnel: w306 -> [_ w323]
                  tunnel: w304 -> [w313 w319]
                  tunnel: [w313 w319] -> w303
                  frame False {
                  }
                  frame True {
                    n67 = call "Update Graphs_JL.vi"("Select Graph"="Select Graph", "appended array"=w323, "ERD Graph  Ind 2"=w324, "Error In"=w327) -> ("All Loads"=→"All Loads":u16[][], "Inlet Thermistor"=→"Inlet Thermistor":u16, "Raw Moisture"=→"Raw Moisture":u16, "Filtered Moisture"=→"Filtered Moisture":u16, "Outlet Thermistor"=→"Outlet Thermistor":u16, "ERD 3"=→"ERD 3":dbl, "ERD 2"=→"ERD 2":dbl, "ERD 1"=→"ERD 1":dbl, "Error Out"=w326:errorcluster)  [unwired: 3 in]
                    "ERD Graph  Ind" <- w324
                  }
                }
              }
              frame Enabled {
              }
            }
          }
          frame "Log Data" {
            # "TimeStamp"
            # "Append With Fault Log Data"
            n68 = Unbundle By Name(w352) -> ("CSV File String Arrays.ERD Name Array"=w350:string[], "CSV File String Arrays.ERD Number Array"=w334:string[], "CSV File String Arrays.ERD Converted String Data"=w339:string[])
            n69 = call "Write_Header_FGV.vi"("Action"=enum16{"Get", "Set"}."Get", "Error In"=w357) -> ("Write Header ? Out"=w340:bool, "Error Out"=w345:errorcluster)  [unwired: 12 in]
            n70 = case shown="True" w340 {
              tunnel: w350 -> [w362 _]
              tunnel: w353 -> [w368 w374]
              tunnel: [w367 w374] -> w338
              tunnel: w352 -> [w363 _]
              tunnel: w334 -> [w361 _]
              frame True {
                # "Write Header"
                n71 = call "Build_Header_RT.vi"("All_Bundled_Data_Brass"=w363, "ERD Number Array In"=w361, "ERD Name Array In"=w362) -> ("ERD Name Array out 2"=w360:string[][])  [unwired: 8 in]
                n72 = Array Size(array=w360) -> (size(s)=w366:i32[])
                n73 = Index Array(array=w366, index=1) -> (element=w364:i32)
                n74 = for {
                  N: w364 -> [_]
                  tunnel: w368 -> [w373]
                  tunnel: [w372] -> w367
                  tunnel: w360 -> [w371]
                  i -> [w370]
                  n75 = Index Array(array=w371, index (row)=w370) -> (element=w369:string[])  [unwired: 1 in]
                  n76 = call "Write _To_CSV_File.vi"("Refnum In"=w373, "ERD Name"=w369) -> ("Refnum Out"=w372:refnum<file>)  [unwired: 15 in, 2 out]
                }
              }
              frame False {
              }
            }
            n77 = call "TimeStamp to String Array.vi"("String Array In"=w339) -> ("String Array Out"=w337:string[])  [unwired: 10 in]
            n78 = Unbundle By Name(w352) -> ("Fault Table Array"=w341:T34)
            n79 = call "Faults_To_String_Array.vi"("Write Header ?"=w340, "Fault Table Entry"=w341, "Error In"=w345) -> ("Fault Header String Array"=w336:string[], "Fault ERD Number String Array"=w335:string[], "Fault Data String Array"=w344:string[], "Error Out"=w342:errorcluster)  [unwired: 13 in]
            n80 = Insert Into Array(array=w337, new element=w344) -> (w343:string[])  [unwired: 1 in]
            n81 = call "Write _To_CSV_File.vi"("Refnum In"=w338, "ERD Name"=w336, "ERD Number"=w335, "ERD Data"=w343, "Error In"=w342) -> ("Refnum Out"=w358:refnum<file>, "Error Out"=w347:errorcluster)  [unwired: 12 in, 1 out]
            n82 = call "Write_Header_FGV.vi"("Write Header ? In"=FALSE, "Action"=enum16{"Get", "Set"}."Set", "Error In"=w347) -> ("Error Out"=w356:errorcluster)  [unwired: 11 in, 1 out]
          }
          frame "Pause" {
            n83 = Wait Until Next ms Multiple(millisecond multiple="Pause(mls)") -> ()  [unwired: 1 out]
          }
          frame "Shutdown" {
          }
        }
        n84 = call "Error_Control.vi"("Error In"=w191) -> ("Error Out"=w193:errorcluster)  [unwired: 14 in]
      }
      n85 = while "UI Loop" {
        shift-right: [w685] -> w135
        shift-left: w103 -> [w679]
        shift-right: [w687] -> w134
        shift-left: _ -> [_]
        tunnel: w61 -> [w686]
        tunnel: w102 -> [w676]
        tunnel: w65 -> [w675]
        tunnel: w48 -> [w674]
        stop <- w684 stop-if-true
        # "UI Loop"
        n86 = call "FGV_GEA2_Ref.vi"("Action"=enum16{"Set Ref", "Get Ref"}."Get Ref", "Error In"=w679) -> ("GEA2 Reference Out"=w678:refnum<k24>, "Error Out"=w680:errorcluster)  [unwired: 12 in]
        n87 = event shown="[21] \"Get Cycle Data\": Value Change" {
          selector: w686 -> [_ _ _ _ _ _ _ _ _ _ _ _ _ _ _ _ _ _ _ _ _ _ _ _ _ _ _ _]
          dyn-events: _ -> [_ _ _ _ _ _ _ _ _ _ _ _ _ _ _ _ _ _ _ _ _ _ _ _ _ _ _ _]
          timeout: 50 -> [_ _ _ _ _ _ _ _ _ _ _ _ _ _ _ _ _ _ _ _ _ _ _ _ _ _ _ _]
          tunnel: [w690 w698 w712 w733 w734 w738 w745 w760 w778 w821 w874 w880 w892 w902 _ w917 w961 w1041 w1048 w1063 w1095 w1112 w1141 w1151 w1164 w1175 _ w1232] -> w683
          tunnel: w680 -> [w691 w700 w715 w730 w734 w739 w744 w759 w786 w826 w879 w890 w896 w903 w908 w914 w963 w1039 w1049 w1064 w1096 w1109 w1142 w1159 w1164 w1182 w1188 w1234]
          tunnel: [_ _ _ _ _ _ _ _ _ _ _ _ _ _ _ _ _ _ _ _ _ _ _ TRUE _ _ _ _] -> w684
          tunnel: w678 -> [w692 w701 w714 w732 w735 w742 w748 _ w787 w827 w878 w889 _ w901 _ w926 w964 _ w1046 w1061 w1099 w1110 _ w1162 w1165 w1181 w1189 w1233]
          tunnel: [w693 w699 w713 w732 w735 w743 w749 _ _ _ _ w888 _ w901 _ _ w960 _ w1047 w1062 w1097 w1111 _ w1162 w1165 w1176 _ w1231] -> w687
          tunnel: "GEA Inputs" -> [_ _ _ _ _ w741 w747 _ _ _ _ _ _ _ _ _ w965 _ w1045 w1065 w1098 w1113 _ _ _ _ w1190 _]
          tunnel: w676 -> [_ _ _ _ _ _ _ _ w783 w825 _ _ _ _ _ w911 _ _ _ _ _ _ _ _ _ _ _ _]
          tunnel: w675 -> [_ _ _ _ _ _ _ _ w777 w822 w873 _ _ _ _ w912 _ w1037 _ _ _ _ w1139 _ _ _ _ _]
          tunnel: w674 -> [_ _ _ _ _ _ _ _ _ _ _ _ _ _ _ _ _ _ _ _ _ _ _ _ _ _ _ _]
          tunnel: "Enum" -> [_ w694 w711 _ _ _ _ _ _ _ _ _ _ _ _ _ _ _ _ _ _ _ _ _ _ _ _ _]
          event "Send Button": Value Change {
            # "GEA2 Tab"
            n88 = event-data() -> ()  [unwired: 1 in, 1 out]
            n89 = call "GEA2 Send and Receive Message.vi"("GEA2 Reference In"=w692, "Input Data"="GEA2 Send", "Error In"=w691) -> ("GEA2 Reference Out"=w693:refnum<k24>, "Converted Data Out"=→"Converted Data Out":T14, "Error Out"=w690:errorcluster)  [unwired: 9 in, 1 out]
          }
          event "Entry Botloader": Value Change {
            n90 = event-data() -> ()  [unwired: 1 in, 1 out]
            n91 = case shown="\"All\", Default" w694 {
              tunnel: T13 {"Source"=229, "Destination"=2, "Command"=221, "Message"="07"} ("GEA2 Send") -> [w703 w707 w708]
              tunnel: [w702 w705 w709] -> w695
              frame "All", Default {
                n92 = Bundle By Name(cluster=w703, "Destination"=u8 255) -> (w702:T13)
              }
              frame "MC" {
                n93 = Bundle By Name(cluster=w707, "Destination"=u8 192) -> (w705:T13)
              }
              frame "UI" {
                n94 = Bundle By Name(cluster=w708, "Destination"=u8 37) -> (w709:T13)
              }
            }
            n95 = call "GEA2 Send and Receive Message.vi"("GEA2 Reference In"=w701, "Input Data"=w695, "Error In"=w700) -> ("GEA2 Reference Out"=w699:refnum<k24>, "Converted Data Out"=w697:T14, "Error Out"=w698:errorcluster)  [unwired: 9 in, 1 out]
            n96 = Unbundle By Name(w697) -> ()  [unwired: 1 out]
          }
          event "Exit Botloader": Value Change {
            n97 = event-data() -> ()  [unwired: 1 in, 1 out]
            n98 = case shown="\"MC\"" w711 {
              tunnel: T13 {"Source"=229, "Destination"=2, "Command"=221, "Message"="F4 01"} ("GEA2 Send") -> [w719 w723 w724]
              tunnel: [w718 w721 w725] -> w716
              frame "All", Default {
                n99 = Bundle By Name(cluster=w719, "Destination"=u8 255) -> (w718:T13)
              }
              frame "MC" {
                n100 = Bundle By Name(cluster=w723, "Destination"=u8 192) -> (w721:T13)
              }
              frame "UI" {
                n101 = Bundle By Name(cluster=w724, "Destination"=u8 37) -> (w725:T13)
              }
            }
            n102 = call "GEA2 Send and Receive Message.vi"("GEA2 Reference In"=w714, "Input Data"=w716, "Error In"=w715) -> ("GEA2 Reference Out"=w713:refnum<k24>, "Error Out"=w712:errorcluster)  [unwired: 9 in, 2 out]
          }
          event "Clear": Value Change {
            w727 = T40 {"Data"=variant, "State"=enum."Clear"} ("element")
            # "GEA2 Tab"
            n103 = event-data() -> ()  [unwired: 1 in, 6 out]
            n104 = Obtain Queue(name (unnamed)="GEA2", element data type=w727, error in (no error)=w730) -> (queue out=w728:refnum<queue>, error out=w731:errorcluster)  [unwired: 2 in, 1 out]
            n105 = Enqueue Element(queue=w728, element=w727, error in (no error)=w731) -> (error out=w733:errorcluster)  [unwired: 1 in, 2 out]
          }
          event Timeout {
            # "Must have timeout case to give GEA2 FGV a chance to update\nthe GEA2 reference. Otherwise, when we receive an event it may\nbe using a reference that is no longer valid."
            n106 = event-data() -> ()  [unwired: 1 in, 3 out]
          }
          event "Write ERD": Value Change {
            # "Read/Write ERDs Tab"
            n107 = event-data() -> ()  [unwired: 1 in, 1 out]
            n108 = call "GEA3 Write ERD (Rev 2 API) Multiple Messages.vi"("GEA2 Reference In"=w742, "# of Tries"=2 ("Retry Count"), "GEA Inputs"=w741, "Write ERD List"="Write ERD List", "Error In"=w739, "Verify ERD Response?"=TRUE) -> ("GEA2 Reference Out"=w743:refnum<k24>, "Error Out"=w738:errorcluster)  [unwired: 7 in, 1 out]
          }
          event "Read ERD": Value Change {
            # "Read/Write ERDs tab"
            n109 = event-data() -> ()  [unwired: 1 in, 6 out]
            n110 = call "GEA3 Read ERD (Rev 2 API) Multiple Messages.vi"("GEA2 Reference In"=w748, "Retry Count"=2, "GEA Inputs"=w747, "Read ERD List"="Read ERD List", "Error In"=w744, "Verify ERD Response?"=TRUE) -> ("GEA2 Reference Out"=w749:refnum<k24>, "ERD Data Out"=→"Read ERD Data Out":cluster{"ERD Number":u16, "Data":string}[], "Error Out"=w745:errorcluster)  [unwired: 6 in, 1 out]
          }
          event "UI Launch": Value Change {
            # "Main"
            n111 = event-data() -> ()  [unwired: 1 in, 6 out]
            n112 = call "HEUI_Running_FGV.vi"("Action"=enum16{"Get", "Set"}."Get", "Error In"=w759) -> ("Running?"=w756:bool, "Error Out"=w758:errorcluster)  [unwired: 12 in]
            n113 = Current VI's Path() -> (path=w754:path)
            n114 = Strip Path(path=w754) -> (stripped path=w755:path)  [unwired: 1 out]
            n115 = case shown="False" w756 {
              tunnel: w758 -> [w770 w772]
              tunnel: [w769 w772] -> w760
              tunnel: w755 -> [w762 _]
              tunnel: "UI Launch" -> [_ _]
              frame False {
                w771 = 128  # options
                n116 = Build Path(base path=w762, name or relative path="JLMainUI.vi") -> (appended path=w767:path)
                n117 = Open VI Reference(type specifier VI Refnum (for type only)=refnum<vi> refnum, vi path=w767, options=w771, error in (no error)=w770) -> (vi reference=w764:refnum<vi>, error out=w766:errorcluster)  [unwired: 2 in]
                n118 = call-by-ref "Start Asynchronous Call"(reference=w764, error in=w766) -> (reference out=w763:refnum<vi>, error out=w765:errorcluster)  [unwired: 10 in, 2 out]
                n119 = Close Reference(reference=w763, error in (no error)=w765) -> (error out=w769:errorcluster)
              }
              frame True {
              }
            }
          }
          event Value Change {
            (unwired) "ERD Loop" ("name (unnamed)")
            w779 = TRUE ("Blinking")
            # "GEA2 Tab"
            n120 = event-data() -> ()  [unwired: 1 in, 1 out]
            n121 = Generate User Event(user event=w783, event data cluster=TRUE ("event data"), error in=w786) -> (error out=w784:errorcluster)  [unwired: 1 in, 1 out]
            n122 = property on="Program Ind" class="Bool (strict)"(error in=w784, "Value"=w779, "Blinking"=w779) -> (error out=w780:errorcluster)  [unwired: 1 in, 1 out]
            n123 = Enqueue Element(queue=w777, element=T38 {"Data"=variant, "State"=enum."Pause"} ("Data"), error in (no error)=w780) -> (error out=w782:errorcluster)  [unwired: 1 in, 2 out]
            n124 = property on="GEA2 Send" class="Clust (strict)"() -> ("Value"=w775:T13)  [unwired: 2 in, 2 out]
            n125 = Unbundle By Name("Programming") -> ("File Path"=w790:path)
            n126 = call "Time Delay3"("error in (no error)"=w782, "Delay Time (s)"=2.0) -> ("error out"=w781:errorcluster)  [unwired: 9 in]
            n127 = Unbundle By Name(w775) -> ("Source"=w774:u8, "Destination"=w773:u8)
            n128 = Not Equal?(x=w790, y=path "") -> (x != y?=w789:bool)
            n129 = case shown="True" w789 {
              tunnel: w781 -> [w793 w798]
              tunnel: [w793 w805] -> w778
              tunnel: w790 -> [_ w810]
              tunnel: w787 -> [_ w806]
              tunnel: w774 -> [_ w795]
              tunnel: w773 -> [_ w794]
              frame False {
              }
              frame True {
                w796 = T12 9 items=["ImageRejected", "BoardNotFound", "UnableToGetGeaConfiguration", "WriteToFlashNotAllowed", "ImageDownloadedSuccessfully", "ImagePresent", "WriteToFlashFailed", "EraseFailed", "CrcFailed", ""] ("Result")
                w804 = FALSE ("Blinking")
                n130 = property on="Result" class="Ring (strict)"(error in=w798, "Value"=w796) -> (error out=w797:errorcluster)  [unwired: 1 in, 1 out]
                n131 = property on="Board Index" class="DigNum (strict)"(error in=w798, "DisabledEnum"=T41."Disabled and Grayed Out" ("Disabled")) -> ()  [unwired: 1 in, 2 out]
                n132 = call "GEA2 Flash APL.vi"("GEA2 Reference In"=w806, "Force Update?"=TRUE, "Source Address"=w795, "Destination Address"=w794, "File Path"=w810, "Error In"=w797, "Broadcast"=TRUE, "Reset?"=FALSE ("Reset Board?")) -> ("Result"=w799:i32, "Error Out"=w801:errorcluster)  [unwired: 3 in, 3 out]
                n133 = property on="Result" class="Ring (strict)"(error in=w801, "Value"=w799) -> (error out=w800:errorcluster)  [unwired: 1 in, 1 out]
                n134 = property on="Board Index" class="DigNum (strict)"(error in=w801, "DisabledEnum"=T41."Enabled" ("Disabled")) -> ()  [unwired: 1 in, 2 out]
                n135 = property on="Program Ind" class="Bool (strict)"(error in=w800, "Value"=w804, "Blinking"=w804) -> (error out=w805:errorcluster)  [unwired: 1 in, 1 out]
              }
            }
          }
          event "Flash Latest": Value Change {
            (unwired) "ERD Loop" ("name (unnamed)")
            w816 = TRUE ("Blinking")
            (unwired) FALSE ("Data On")
            # "GEA2 Tab"
            n136 = event-data() -> ()  [unwired: 1 in, 6 out]
            n137 = Generate User Event(user event=w825, event data cluster=TRUE ("event data"), error in=w826) -> (error out=w818:errorcluster)  [unwired: 1 in, 1 out]
            n138 = property on="Program Ind" class="Bool (strict)"(error in=w818, "Value"=w816, "Blinking"=w816) -> (error out=w817:errorcluster)  [unwired: 1 in, 1 out]
            n139 = Enqueue Element(queue=w822, element=T38 {"Data"=variant, "State"=enum."Pause"} ("Data"), error in (no error)=w817) -> (error out=w824:errorcluster)  [unwired: 1 in, 2 out]
            n140 = call "JL_Get_Latest_Build_From_Artifactory.vi"("Repository"="CIBuild") -> ("Output Path"=w811:path)  [unwired: 12 in, 2 out]
            n141 = call "Time Delay2"("error in (no error)"=w824, "Delay Time (s)"=3.0) -> ("error out"=w823:errorcluster)  [unwired: 9 in]
            n142 = Not Equal?(x=w811, y=path "") -> (x != y?=w829:bool)
            n143 = case shown="True" w829 {
              tunnel: w823 -> [w832 w856]
              tunnel: [w832 w844] -> w814
              tunnel: w827 -> [_ w857]
              tunnel: w811 -> [_ w833]
              frame False {
              }
              frame True {
                w836 = T12 9 items=["ImageRejected", "BoardNotFound", "UnableToGetGeaConfiguration", "WriteToFlashNotAllowed", "ImageDownloadedSuccessfully", "ImagePresent", "WriteToFlashFailed", "EraseFailed", "CrcFailed", ""] ("Result")
                w843 = FALSE ("Blinking")
                n144 = call "JL_APLPath.vi"("Error In"=w856, "APL Search String"=T42."UI Application APL", "Folder Path"=w833) -> ("Error Out"=w855:errorcluster, "File Path"=w854:path)  [unwired: 5 in, 2 out]
                n145 = call "GEA2 Flash APL.vi"("GEA2 Reference In"=w857, "Force Update?"=TRUE, "Source Address"=u8 228, "Destination Address"=u8 36, "File Path"=w854, "Error In"=w855, "Broadcast"=TRUE, "Reset?"=FALSE ("Reset Board?")) -> ("GEA2 Reference Out"=w846:refnum<k24>, "Result"=w840:i32, "Error Out"=w842:errorcluster)  [unwired: 3 in, 2 out]
                n146 = property on="Board Index" class="DigNum (strict)"(error in=w856, "DisabledEnum"=T41."Disabled and Grayed Out" ("Disabled")) -> (error out=w839:errorcluster)  [unwired: 1 in, 1 out]
                n147 = property on="Result" class="Ring (strict)"(error in=w842, "Value"=w840) -> (error out=w841:errorcluster)  [unwired: 1 in, 1 out]
                n148 = property on="Result" class="Ring (strict)"(error in=w839, "Value"=w836) -> ()  [unwired: 1 in, 2 out]
                n149 = call "JL_APLPath.vi"("Error In"=w841, "APL Search String"=T42."UI Parametric APL", "Folder Path"=w833) -> ("Error Out"=w852:errorcluster, "File Path"=w853:path)  [unwired: 5 in, 2 out]
                n150 = call "GEA2 Flash APL.vi"("GEA2 Reference In"=w846, "Force Update?"=TRUE, "Source Address"=u8 228, "Destination Address"=u8 36, "File Path"=w853, "Error In"=w852, "Broadcast"=TRUE, "Reset?"=TRUE ("Reset Board?")) -> ("Result"=w837:i32, "Error Out"=w845:errorcluster)  [unwired: 3 in, 3 out]
                n151 = property on="Board Index" class="DigNum (strict)"(error in=w845, "DisabledEnum"=T41."Enabled" ("Disabled")) -> (error out=w838:errorcluster)  [unwired: 1 in, 1 out]
                n152 = property on="Program Ind" class="Bool (strict)"(error in=w845, "Value"=w843, "Blinking"=w843) -> (error out=w844:errorcluster)  [unwired: 1 in, 1 out]
                n153 = property on="Result" class="Ring (strict)"(error in=w838, "Value"=w837) -> ()  [unwired: 1 in, 2 out]
              }
            }
            n154 = call "Time Delay4"("error in (no error)"=w814, "Delay Time (s)"=3.0) -> ("error out"=w813:errorcluster)  [unwired: 9 in]
            n155 = Enqueue Element(queue=w822, element=T38 {"Data"=variant, "State"=enum."Init"} ("Data"), error in (no error)=w813) -> (error out=w821:errorcluster)  [unwired: 1 in, 2 out]
          }
          event Value Change {
            # "GEA2 TAB"
            n156 = event-data() -> ()  [unwired: 1 in, 6 out]
            n157 = property on="GEA2 Send" class="Clust (strict)"() -> ("Value"=w868:T13)  [unwired: 2 in, 2 out]
            n158 = Unbundle By Name(w868) -> ("Source"=w867:u8)
            n159 = Bundle By Name(cluster=T13 {"Source"=228, "Destination"=2, "Command"=221, "Message"="F401"} ("Input Data"), "Source"=w867, "Destination"=u8 255, "Command"=u8 221, "Message"="F401") -> (w871:T13)
            n160 = call "GEA2 Send Message.vi"("GEA2 Reference In"=w878, "Input Data"=w871, "Error In"=w879) -> ("Error Out"=w865:errorcluster)  [unwired: 11 in, 1 out]
            n161 = call "Time Delay5"("error in (no error)"=w865, "Delay Time (s)"=3.0) -> ("error out"=w875:errorcluster)  [unwired: 9 in]
            n162 = Enqueue Element(queue=w873, element=T38 {"Data"=variant, "State"=enum."Init"} ("Data"), error in (no error)=w875) -> (error out=w874:errorcluster)  [unwired: 1 in, 2 out]
          }
          event Value Change {
            # "GEA2 Tab"
            n163 = event-data() -> ()  [unwired: 1 in, 6 out]
            n164 = property on="GEA2 Send" class="Clust (strict)"() -> ("Value"=w887:T13)  [unwired: 2 in, 2 out]
            n165 = Unbundle By Name(w887) -> ("Source"=w883:u8, "Destination"=w882:u8)
            n166 = Bundle By Name(cluster=T13 {"Source"=228, "Destination"=2, "Command"=221, "Message"="F401"} ("Input Data"), "Source"=w883, "Destination"=w882, "Command"=u8 221, "Message"="07") -> (w881:T13)
            n167 = call "GEA2 Send Message.vi"("GEA2 Reference In"=w889, "Input Data"=w881, "Error In"=w890) -> ("GEA2 Reference Out"=w888:refnum<k24>, "Error Out"=w880:errorcluster)  [unwired: 11 in]
          }
          event "Save Log": Value Change {
            # "GEA2 Tab"
            n168 = event-data() -> ()  [unwired: 1 in, 6 out]
            n169 = property on="GEA2 Log" class="Str"(error in=w896) -> (error out=w898:errorcluster, "Value"=w897:string)  [unwired: 1 in, 1 out]
            n170 = Write to Text File(prompt (Choose or enter file path)="Choose filename and path to save txt file to ", text=w897, error in=w898) -> (refnum out=w895:refnum<file>, error out=w894:errorcluster)  [unwired: 1 in, 1 out]
            n171 = Close File(refnum=w895, error in=w894) -> (error out=w893:errorcluster)  [unwired: 1 out]
            n172 = call <vilib>:"Clear Errors.vi"("error in (no error)"=w893, "specific error code to clear (0: all)"=43) -> ("error out"=w892:errorcluster)  [unwired: 4 in, 1 out]
          }
          event "Desired FilteredMoisture": Value Change {
            # "MoistureSensorReset"
            # "DAQ Tab"
            n173 = event-data() -> ()  [unwired: 1 in, 6 out]
            n174 = call "MoistureSensorReset.vi"("GEA2 Reference In"=w901, "Error In"=w903) -> ("Error Out"=w900:errorcluster)  [unwired: 10 in, 3 out]
            n175 = call "JL_Scaling Factor.vi"("Error"=w900, "Scalling"="Scalling", "Scaling Type"="Init/Scale", "Desired Value Out"="Desired FilteredMoisture") -> ("Error Out"=w902:errorcluster, "Analog Value Out"=w907:dbl)  [unwired: 5 in, 1 out]
            n176 = property on="Moisture (V)" class="Slide (strict)"("Value"=w907) -> ()  [unwired: 2 in, 2 out]
          }
          event "Model": Value Change {
            # "No esta activado"
            n177 = event-data() -> ("NewVal"=w910:enum16{"Estar Centauro", "GFL"})  [unwired: 1 in, 5 out]
            n178 = call "Set Get Model.vi"("Error In"=w908, "Action"=enum16{"Set Model", "Get Model"}."Set Model", "Model"=w910) -> ()  [unwired: 7 in, 2 out]
          }
          event "Run Script": Value Change {
            w938 = T27 {"Overall Script File Progress"=0.0, "Current Script Progress"=0.0, "Script"="", "Test"="", "Elapsed time (s)"=0.0, "Done?"=FALSE}  # Script Info
            w930 = T13 {"Source"=228, "Destination"=35, "Command"=1, "Message"=""}  # Version Query (for log header)
            # "Scripting Tab"
            n179 = event-data() -> ()  [unwired: 1 in, 6 out]
            n180 = Generate User Event(user event=w911, event data cluster=TRUE ("event data"), error in=w914) -> (error out=w915:errorcluster)  [unwired: 1 in, 1 out]
            n181 = Enqueue Element(queue=w912, element=T38 {"Data"=variant, "State"=enum."Pause"} ("Data"), error in (no error)=w915) -> (error out=w913:errorcluster)  [unwired: 1 in, 2 out]
            n182 = Obtain Queue(name (unnamed)="Script_Stop", element data type=FALSE, error in (no error)=w913) -> (queue out=w934:refnum<queue>, error out=w937:errorcluster)  [unwired: 2 in, 1 out]
            n183 = Obtain Queue(name (unnamed)="Script_Info", element data type=w938, error in (no error)=w937) -> (queue out=w940:refnum<queue>, error out=w931:errorcluster)  [unwired: 2 in, 1 out]
            n184 = while {
              tunnel: w940 -> [w952]
              shift-right: [w945] -> w928
              shift-left: w931 -> [w948]
              tunnel: [w951] -> w939
              tunnel: w934 -> [w949]
              tunnel: [w944] -> w932
              stop <- w950 stop-if-true
              n185 = Dequeue Element(queue=w952, error in (no error)=w948) -> (queue out=w951:refnum<queue>, element=w943:T27, error out=w947:errorcluster)  [unwired: 1 in, 1 out]
              "Script Info" <- w943
              n186 = Unbundle By Name(w943) -> ("Done?"=w950:bool)
              n187 = case shown="False" "stop script" {
                selector: "stop script" -> [_ w955]
                tunnel: w949 -> [w954 w959]
                tunnel: w948 -> [w953 w958]
                tunnel: [w953 w957] -> w946
                tunnel: [w954 w956] -> w944
                frame False {
                }
                frame True {
                  n188 = Enqueue Element(queue=w959, element=w955, error in (no error)=w958) -> (queue out=w956:refnum<queue>, error out=w957:errorcluster)  [unwired: 1 in, 1 out]
                }
              }
              n189 = Merge Errors(w946, w947) -> (w945:errorcluster)
            }
            n190 = call "GEA2 Script Test SLB.vi"("GEA2 Reference In"=w926, "Version Query (for log header)"=w930, "Enqueue Sends?"=TRUE, "Standalone"=FALSE, "Script path"="Script Path", "Log File Path (empty for prompt)"="Script Log Path", "Error In"=w931) -> ("Pass/Fail?"=→"Script Pass/Fail?":bool, "Report Text"=→"Script Report Text":string, "Error Out"=→"Script Error Out":errorcluster)  [unwired: 5 in, 1 out]
            n191 = Release Queue(queue=w939, error in (no error)=w928) -> (error out=w933:errorcluster)  [unwired: 1 in, 2 out]
            n192 = Release Queue(queue=w932, error in (no error)=w933) -> (error out=w918:errorcluster)  [unwired: 1 in, 2 out]
            n193 = Enqueue Element(queue=w912, element=T38 {"Data"=variant, "State"=enum."Init"} ("Data"), error in (no error)=w918) -> (error out=w917:errorcluster)  [unwired: 1 in, 2 out]
          }
          event "LED Control.ALL LEDs ON", "LED Control.ALL LEDs OFF", "LED Control.Reset LEDs": Value Change {
            # "Load Control Tab"
            n194 = event-data() -> ("CtlRef"=w962:refnum<vi>)  [unwired: 1 in, 5 out]
            n195 = property class="Bool"(reference=w962, error in=w963) -> (reference out=w967:refnum<vi>, error out=w968:errorcluster, "Label.Text"=w966:string)
            n196 = Close Reference(reference=w967, error in (no error)=w968) -> (error out=w969:errorcluster)
            n197 = case shown="\"ALL LEDs ON\"" w966 {
              tunnel: w969 -> [w974 w992 w1010]
              tunnel: w965 -> [w975 w993 w1008]
              tunnel: w964 -> [w973 w991 w1009]
              tunnel: [w972 w990 w1007] -> w960
              tunnel: [w971 w989 w1006] -> w961
              frame "ALL LEDs ON" {
                w985 = T5 {"ERD Number"=61724, "Data Type"=enum."string", "Data"=""}  # ERD Read Data In
                n198 = Concatenate Strings("0101FFFFFFFFFFFFFFFFFFFF" ("string")) -> (w986:string)
                n199 = Bundle By Name(cluster=w985, "Data"=w986) -> (w984:T5)
                n200 = Build Array(w984) -> (w977:T5[])
                n201 = call "Convert Write ERD List to Message.vi"("GEA Inputs"=w975, "Write ERD List"=w977, "Error In"=w974) -> ("GEA Message"=w979:T13, "Error Out"=w980:errorcluster)  [unwired: 11 in]
                n202 = call "GEA2MessageFormatter.vi"("Prefix(Send/Recv)"="SEND", "GEA2 Data In"=w979, "Error In"=w980) -> ("Output String"=w981:string, "Error Out"=w982:errorcluster)  [unwired: 11 in]
                n203 = call "GExplorer_Queue_GEA2.vi"("Output String"=w981, "error in (no error)"=w982) -> ("error out"=w978:errorcluster)  [unwired: 13 in]
                n204 = call "GEA2 Write ERD.vi"("GEA2 Reference In"=w973, "GEA Inputs"=w975, "Write ERD List"=w977, "Error In"=w978, "Verify ERD Response?"=TRUE) -> ("GEA2 Reference Out"=w972:refnum<k24>, "Error Out"=w971:errorcluster)  [unwired: 8 in, 1 out]
              }
              frame "ALL LEDs OFF" {
                n205 = Concatenate Strings("010100000000000000000000" ("string")) -> (w1003:string)
                n206 = Bundle By Name(cluster=T5 {"ERD Number"=61724, "Data Type"=enum."string", "Data"=""} ("ERD Read Data In"), "Data"=w1003) -> (w1002:T5)
                n207 = Build Array(w1002) -> (w995:T5[])
                n208 = call "Convert Write ERD List to Message.vi"("GEA Inputs"=w993, "Write ERD List"=w995, "Error In"=w992) -> ("GEA Message"=w997:T13, "Error Out"=w998:errorcluster)  [unwired: 11 in]
                n209 = call "GEA2MessageFormatter.vi"("Prefix(Send/Recv)"="SEND", "GEA2 Data In"=w997, "Error In"=w998) -> ("Output String"=w999:string, "Error Out"=w1000:errorcluster)  [unwired: 11 in]
                n210 = call "GExplorer_Queue_GEA2.vi"("Output String"=w999, "error in (no error)"=w1000) -> ("error out"=w996:errorcluster)  [unwired: 13 in]
                n211 = call "GEA2 Write ERD.vi"("GEA2 Reference In"=w991, "GEA Inputs"=w993, "Write ERD List"=w995, "Error In"=w996, "Verify ERD Response?"=TRUE) -> ("GEA2 Reference Out"=w990:refnum<k24>, "Error Out"=w989:errorcluster)  [unwired: 8 in, 1 out]
              }
              frame "Reset LEDS", Default {
                w1022 = T5 {"ERD Number"=61724, "Data Type"=enum."string", "Data"=""}  # ERD Read Data In
                n212 = Concatenate Strings("010100000000000000000000" ("string")) -> (w1023:string)
                n213 = Bundle By Name(cluster=w1022, "Data"=w1023) -> (w1021:T5)
                n214 = Build Array(w1021) -> (w1014:T5[])
                n215 = call "Convert Write ERD List to Message.vi"("GEA Inputs"=w1008, "Write ERD List"=w1014, "Error In"=w1010) -> ("GEA Message"=w1016:T13, "Error Out"=w1017:errorcluster)  [unwired: 11 in]
                n216 = call "GEA2MessageFormatter.vi"("Prefix(Send/Recv)"="SEND", "GEA2 Data In"=w1016, "Error In"=w1017) -> ("Output String"=w1018:string, "Error Out"=w1019:errorcluster)  [unwired: 11 in]
                n217 = call "GExplorer_Queue_GEA2.vi"("Output String"=w1018, "error in (no error)"=w1019) -> ("error out"=w1015:errorcluster)  [unwired: 13 in]
                n218 = call "GEA2 Write ERD.vi"("GEA2 Reference In"=w1009, "GEA Inputs"=w1008, "Write ERD List"=w1014, "Error In"=w1015, "Verify ERD Response?"=TRUE) -> ("GEA2 Reference Out"=w1011:refnum<k24>, "Error Out"=w1012:errorcluster)  [unwired: 8 in, 1 out]
                n219 = Concatenate Strings("000000000000000000000000" ("string")) -> (w1034:string)
                n220 = Bundle By Name(cluster=T5 {"ERD Number"=61724, "Data Type"=enum."string", "Data"=""} ("ERD Read Data In"), "Data"=w1034) -> (w1032:T5)
                n221 = Build Array(w1032) -> (w1025:T5[])
                n222 = call "Convert Write ERD List to Message.vi"("GEA Inputs"=w1008, "Write ERD List"=w1025, "Error In"=w1012) -> ("GEA Message"=w1027:T13, "Error Out"=w1028:errorcluster)  [unwired: 11 in]
                n223 = call "GEA2MessageFormatter.vi"("Prefix(Send/Recv)"="SEND", "GEA2 Data In"=w1027, "Error In"=w1028) -> ("Output String"=w1029:string, "Error Out"=w1030:errorcluster)  [unwired: 11 in]
                n224 = call "GExplorer_Queue_GEA2.vi"("Output String"=w1029, "error in (no error)"=w1030) -> ("error out"=w1026:errorcluster)  [unwired: 13 in]
                n225 = call "GEA2 Write ERD.vi"("GEA2 Reference In"=w1011, "GEA Inputs"=w1008, "Write ERD List"=w1025, "Error In"=w1026, "Verify ERD Response?"=TRUE) -> ("GEA2 Reference Out"=w1007:refnum<k24>, "Error Out"=w1006:errorcluster)  [unwired: 8 in, 1 out]
              }
            }
          }
          event Value Change {
            # "ERD List"
            n226 = event-data() -> ()  [unwired: 1 in, 6 out]
            n227 = Enqueue Element(queue=w1037, element=T38 {"Data"=variant, "State"=enum."Build ERD Read List"}, error in (no error)=w1039) -> (error out=w1038:errorcluster)  [unwired: 1 in, 2 out]
            n228 = call "Write_Header_FGV.vi"("Write Header ? In"=TRUE, "Action"=enum16{"Get", "Set"}."Set", "Error In"=w1038) -> ("Error Out"=w1041:errorcluster)  [unwired: 11 in, 1 out]
            n229 = call "Select_List.vi"("Load ERD List"="Load ERD List") -> ()  [unwired: 14 in, 1 out]
          }
          event "Clear Fault Seq Buffer": Value Change {
            w1057 = T5 {"ERD Number"=57626, "Data Type"=enum."string", "Data"=""}  # ERD Read Data In
            # "Faults Tab"
            n230 = event-data() -> ()  [unwired: 1 in, 6 out]
            n231 = Bundle By Name(cluster=w1057, "Data"="01") -> (w1056:T5)
            n232 = Build Array(w1056) -> (w1043:T5[])
            n233 = call "Convert Write ERD List to Message.vi"("GEA Inputs"=w1045, "Write ERD List"=w1043, "Error In"=w1049) -> ("GEA Message"=w1052:T13, "Error Out"=w1053:errorcluster)  [unwired: 11 in]
            n234 = call "GEA2MessageFormatter.vi"("Prefix(Send/Recv)"="SEND", "GEA2 Data In"=w1052, "Error In"=w1053) -> ("Output String"=w1054:string, "Error Out"=w1055:errorcluster)  [unwired: 11 in]
            n235 = call "GExplorer_Queue_GEA2.vi"("Output String"=w1054, "error in (no error)"=w1055) -> ("error out"=w1044:errorcluster)  [unwired: 13 in]
            n236 = call "GEA3 Write ERD (Rev 2 API) Multiple Messages.vi"("GEA2 Reference In"=w1046, "GEA Inputs"=w1045, "Write ERD List"=w1043, "Error In"=w1044) -> ("GEA2 Reference Out"=w1047:refnum<k24>, "Error Out"=w1048:errorcluster)  [unwired: 9 in, 1 out]
          }
          event "Get Faults": Value Change {
            # "Faults Tab"
            n237 = event-data() -> ()  [unwired: 1 in, 6 out]
            n238 = call "Main_Decode_V3.vi"("GEA2 Reference In"=w1061, "GEA Inputs"=w1065, "Error In"=w1064) -> ("Fault Table Status"=w1083:T19[], "Major Version"=→"Major Version":u8, "Minor Version"=→"Minor Version":u8, "Fault Table Entries"=w1082:T20[][], "GEA2 Reference Out"=w1072:refnum<k24>, "Diagnostic Entity Manifest"=w1080:T21[], "SnapShot ERD List"=w1070:T4[][], "Fault Sequence Status"=w1073:T19[], "Fault Sequence Entries"=w1081:T18[][], "Error Out"=w1071:errorcluster)  [unwired: 5 in, 2 out]
            n239 = Index Array(array=w1082) -> (element=w1078:T20[])  [unwired: 2 in]
            n240 = Index Array(array=w1083) -> (element=w1059:T19)  [unwired: 1 in]
            "Fault Table Status" <- w1059
            n241 = Index Array(array=w1080) -> (element=→"Diagnostic Entity Manifest":T21)  [unwired: 1 in]
            n242 = Index Array(array=w1081) -> (element=w1075:T18[])  [unwired: 2 in]
            n243 = Index Array(array=w1073) -> (element=w1068:T19)  [unwired: 1 in]
            "Fault Seq Status" <- w1068
            n244 = call "JL_Diag_Filter_Faults.vi"("Filter by Count"="Filter by Count", "Fault Table Entries In"=w1078, "Status"=w1059) -> ("Fault Table Entries Out"=→"Fault Table Entries":T20[], "Fault Set?"=→"Fault Set?":bool)  [unwired: 11 in]
            n245 = call "JL_Diag_Filter_Seq.vi"("Filter by Count"="Filter by Count", "Fault Table Entries In"=w1075, "Status"=w1068) -> ("Fault Table Entries Out"=→"Fault Sequence Entries":T18[])  [unwired: 12 in]
            n246 = Unbundle By Name(w1059) -> ("Count"=w1058:u16)
            n247 = Index Array(array=w1070) -> (element=w1069:T4[])  [unwired: 2 in]
            n248 = for {
              N: w1058 -> [_]
              tunnel: [w1092] -> w1067 mode=indexing
              tunnel: w1065 -> [w1090]
              shift-right: [w1089] -> w1062
              shift-left: w1072 -> [w1091]
              shift-right: [w1087] -> w1063
              shift-left: w1071 -> [w1088]
              tunnel: w1069 -> [w1086] mode=indexing
              tunnel: "Filter by Count" -> [_]
              n249 = call "JL_Parse_Snapshot.vi"("GEA2 Reference In"=w1091, "GEA Inputs"=w1090, "SnapShot Location"=w1086, "Error In"=w1088) -> ("GEA2 Reference Out"=w1089:refnum<k24>, "Fault Snapshot"=w1092:string[], "Error Out"=w1087:errorcluster)  [unwired: 9 in]
            }
            n250 = Transpose 2D Array(2D array=w1067) -> (transposed array=→"Centauro Fault Snapshot":string[][])
          }
          event "Clear Fault Table Buffer": Value Change {
            # "Faults Tab"
            n251 = event-data() -> ()  [unwired: 1 in, 6 out]
            n252 = Bundle By Name(cluster=T5 {"ERD Number"=57604, "Data Type"=enum."string", "Data"=""} ("ERD Read Data In"), "Data"="01") -> (w1102:T5)
            n253 = Build Array(w1102) -> (w1100:T5[])
            n254 = call "GEA3 Write ERD (Rev 2 API) Multiple Messages.vi"("GEA2 Reference In"=w1099, "# of Tries"=u8 3, "Read Timeout (ms)"=u32 250, "GEA Inputs"=w1098, "Write ERD List"=w1100, "Error In"=w1096) -> ("GEA2 Reference Out"=w1097:refnum<k24>, "Error Out"=w1095:errorcluster)  [unwired: 7 in, 1 out]
          }
          event "Get Cycle Data": Value Change {
            w1105 = T4[] [{"ERD Number"=57661, "Data Type"=enum."string"}, {"ERD Number"=57662, "Data Type"=enum."string"}, {"ERD Number"=57663, "Data Type"=enum."string"}, {"ERD Number"=57664, "Data Type"=enum."string"}, {"ERD Number"=57665, "Data Type"=enum."string"}, {"ERD Number"=57666, "Data Type"=enum."string"}, {"ERD Number"=57667, "Data Type"=enum."string"}, {"ERD Number"=57668, "Data Type"=enum."string"}, {"ERD Number"=57669, "Data Type"=enum."string"}, {"ERD Number"=57670, "Data Type"=enum."string"}, {"ERD Number"=57671, "Data Type"=enum."string"}, {"ERD Number"=57672, "Data Type"=enum."string"}, {"ERD Number"=57673, "Data Type"=enum."string"}, {"ERD Number"=57674, "Data Type"=enum."string"}, {"ERD Number"=57675, "Data Type"=enum."string"}, {"ERD Number"=57676, "Data Type"=enum."string"}, {"ERD Number"=57677, "Data Type"=enum."string"}, {"ERD Number"=57678, "Data Type"=enum."string"}, {"ERD Number"=57679, "Data Type"=enum."string"}, {"ERD Number"=57680, "Data Type"=enum."string"}]
            # "E13D"
            # "Faults Tab"
            # "Erd_DiagnosticsCycleHistorySequenceEntry[0:19]"
            # "Erd_ServiceDiagnosticsCycleHistorySequenceStatus"
            n255 = event-data() -> ()  [unwired: 1 in, 1 out]
            n256 = call "GEA2 Read ERD.vi"("GEA2 Reference In"=w1110, "GEA Inputs"=w1113, "Read ERD List"=T4[] [{"ERD Number"=57659, "Data Type"=enum."string"}], "Error In"=w1109) -> ("GEA2 Reference Out"=w1115:refnum<k24>, "ERD Data Out"=w1118:T7[], "Error Out"=w1114:errorcluster)  [unwired: 8 in, 1 out]
            n257 = Index Array(array=w1118) -> (element=w1119:T7)  [unwired: 1 in]
            n258 = Unbundle By Name(w1119) -> ("Data"=w1129:string)
            n259 = call "HexStringToU16.vi"("Input String"=w1129, "Starting Offset"=0) -> ("Number Out"=w1127:u16)  [unwired: 13 in]
            n260 = call "HexStringToU16.vi"("Input String"=w1129, "Starting Offset"=6) -> ("Number Out"=w1130:u16)  [unwired: 13 in]
            n261 = call "HexStringToU16.vi"("Input String"=w1129, "Starting Offset"=12) -> ("Number Out"=w1128:u16)  [unwired: 13 in]
            n262 = Array Size(array=w1105) -> (size(s)=w1121:i32)
            n263 = Select(t=w1130, s="Filter by Status Count", f=w1121) -> (s? t:f=w1120:i32)
            n264 = Bundle By Name(cluster=T19 {"Cur Index"=0, "Count"=0, "Ov Cnt"=0} ("Fault Table Status"), "Cur Index"=w1127, "Count"=w1130, "Ov Cnt"=w1128) -> (→"output cluster":T19)
            n265 = Array Subset(array=w1105, length=w1120) -> (w1117:T4[])  [unwired: 1 in]
            n266 = for {
              shift-right: [w1137] -> w1112
              shift-left: w1114 -> [w1138]
              shift-right: [w1135] -> w1111
              shift-left: w1115 -> [w1136]
              tunnel: w1117 -> [w1134] mode=indexing
              tunnel: w1113 -> [w1133]
              tunnel: [w1132] -> w1108 mode=indexing
              tunnel: [w1131] -> w1104
              n267 = call "JL_Cycle_History_ParseRecord.vi"("Error In"=w1138, "Cycle History ERD"=w1134, "GEA Inputs"=w1133, "GEA2 Reference In"=w1136) -> ("Error Out"=w1137:errorcluster, "Bits"=w1131:i32, "CS2 Dryer"=w1132:string[], "GEA2 Reference Out"=w1135:refnum<k24>)  [unwired: 3 in]
            }
            "Bits" <- w1104
            n268 = Transpose 2D Array(2D array=w1108) -> (transposed array=→"JL Cycle History":string[][])
          }
          event "Data ON": Value Change {
            # "Main"
            n269 = event-data() -> ()  [unwired: 1 in, 6 out]
            n270 = case shown="True" "Data ON" {
              tunnel: w1142 -> [w1145 w1149]
              tunnel: [w1144 w1148] -> w1141
              tunnel: w1139 -> [w1143 w1147]
              frame True {
                n271 = Enqueue Element(queue=w1143, element=T38 {"Data"=variant, "State"=enum."Init"} ("Data"), error in (no error)=w1145) -> (error out=w1144:errorcluster)  [unwired: 1 in, 2 out]
              }
              frame False {
                n272 = Enqueue Element(queue=w1147, element=T38 {"Data"=variant, "State"=enum."Pause"} ("Data"), error in (no error)=w1149) -> (error out=w1148:errorcluster)  [unwired: 1 in, 2 out]
              }
            }
          }
          event "Stop": Value Change; User Event; Panel Close {
            # "Main"
            n273 = event-data() -> ()  [unwired: 1 in, 3 out]
            n274 = call "Control_ERD_Loop.vi"("Command (ERD Loop Control)"=ERD_Loop_Control_Command."Shutdown", "Error In"=w1159) -> ("Error Out"=w1158:errorcluster)  [unwired: 13 in]
            n275 = call "Control_GEA2_Loop.vi"("Command (ERD Loop Control)"=GEA2_Control_Command."Shutdown", "Error In"=w1158) -> ("Error Out"=w1160:errorcluster)  [unwired: 13 in]
            n276 = call "Control_DAQ_Loop.vi"("Command (DAQ Control)"=DAQ_Control_Command."Shutdown", "Error In"=w1160) -> ("Error Out"=w1163:errorcluster)  [unwired: 13 in]
            n277 = call "Control_Cont_Send.vi"("Command (ERD Loop Control)"=GEA2_Control_Command."Shutdown", "Error In"=w1163) -> ("Error Out"=w1152:errorcluster)  [unwired: 13 in]
            n278 = call "Time Delay6"("error in (no error)"=w1152, "Delay Time (s)"=2.0) -> ("error out"=w1151:errorcluster)  [unwired: 9 in]
          }
          event "Tool Version": Value Change {
            # "Version Tab"
            n279 = event-data() -> ()  [unwired: 1 in, 6 out]
            n280 = property class="App"() -> ("App.Kind"=w1166:T46)  [unwired: 2 in, 2 out]
            n281 = case shown="\"invalid app kind\", Default" w1166 {
              tunnel: ["invalid" ("File Version Info") w1169 w1174] -> w1167
              frame "invalid app kind", Default {
              }
              frame "Development System", "Student Edition".."Evaluation" {
                n282 = property class="App"() -> ("App.Version"=w1169:string)  [unwired: 2 in, 2 out]
              }
              frame "Run Time System" {
                n283 = property class="App"() -> ("App.Dir"=w1172:path, "App.Name"=w1173:string)  [unwired: 2 in, 2 out]
                n284 = Build Path(base path=w1172, name or relative path=w1173) -> (appended path=w1171:path)
                n285 = call <vilib>:"FileVersionInfo.vi"("Application Path in"=w1171) -> ("FileVersionInfo Out"=→"FileVersionInfo":T10, "File Version Info"=w1174:string)  [unwired: 7 in, 2 out]
              }
            }
            "LabView/Version Number" <- w1167
          }
          event "Get Wifi Data": Value Change {
            n286 = event-data() -> ()  [unwired: 1 in, 6 out]
            n287 = call "Wifi_Data.vi"("GEA2 Reference In"=w1181, "Error In"=w1182) -> ("Wifi Network State"=→"Wifi Network State":string, "GEA2 Reference Out"=w1176:refnum<k24>, "Mac Address"=→"Mac Address":string, "Wifi Network Name"=→"Wifi Network Name":string, "Wifi Password"=→"Wifi Password":string, "Error Out"=w1175:errorcluster)  [unwired: 8 in]
          }
          event "Turn off Wifi", "Turn on Wifi": Value Change {
            w1184 = T5 {"ERD Number"=61717, "Data Type"=enum."string", "Data"=""} ("ERD Read Data In")
            n288 = event-data() -> ()  [unwired: 1 in, 6 out]
            n289 = case shown="True" "Turn on Wifi" {
              tunnel: w1189 -> [w1212 w1219]
              tunnel: w1188 -> [w1213 w1218]
              tunnel: w1184 -> [_ w1217]
              tunnel: [w1213 w1215] -> w1186
              tunnel: [w1212 w1216] -> w1187
              tunnel: w1190 -> [w1211 w1214]
              tunnel: [w1211 w1214] -> w1185
              frame False {
              }
              frame True {
                n290 = Concatenate Strings("01" ("string")) -> (w1230:string)
                n291 = Bundle By Name(cluster=w1217, "Data"=w1230) -> (w1229:T5)
                n292 = Build Array(w1229) -> (w1220:T5[])
                n293 = call "Convert Write ERD List to Message.vi"("GEA Inputs"=w1214, "Write ERD List"=w1220, "Error In"=w1218) -> ("GEA Message"=w1224:T13, "Error Out"=w1225:errorcluster)  [unwired: 11 in]
                n294 = call "GEA2MessageFormatter.vi"("Prefix(Send/Recv)"="SEND", "GEA2 Data In"=w1224, "Error In"=w1225) -> ("Output String"=w1226:string, "Error Out"=w1227:errorcluster)  [unwired: 11 in]
                n295 = call "GExplorer_Queue_GEA2.vi"("Output String"=w1226, "error in (no error)"=w1227) -> ("error out"=w1223:errorcluster)  [unwired: 13 in]
                n296 = call "GEA2 Write ERD.vi"("GEA2 Reference In"=w1219, "GEA Inputs"=w1214, "Write ERD List"=w1220, "Error In"=w1223, "Verify ERD Response?"=FALSE) -> ("GEA2 Reference Out"=w1216:refnum<k24>, "Error Out"=w1215:errorcluster)  [unwired: 8 in, 1 out]
              }
            }
            n297 = case shown="True" "Turn off Wifi" {
              tunnel: w1187 -> [w1192 w1199]
              tunnel: w1186 -> [w1193 w1198]
              tunnel: [w1193 w1196] -> _
              tunnel: [w1192 w1197] -> _
              tunnel: w1185 -> [_ w1195]
              tunnel: w1184 -> [_ w1194]
              frame False {
              }
              frame True {
                n298 = Concatenate Strings("02" ("string")) -> (w1210:string)
                n299 = Bundle By Name(cluster=w1194, "Data"=w1210) -> (w1209:T5)
                n300 = Build Array(w1209) -> (w1200:T5[])
                n301 = call "Convert Write ERD List to Message.vi"("GEA Inputs"=w1195, "Write ERD List"=w1200, "Error In"=w1198) -> ("GEA Message"=w1204:T13, "Error Out"=w1205:errorcluster)  [unwired: 11 in]
                n302 = call "GEA2MessageFormatter.vi"("Prefix(Send/Recv)"="SEND", "GEA2 Data In"=w1204, "Error In"=w1205) -> ("Output String"=w1206:string, "Error Out"=w1207:errorcluster)  [unwired: 11 in]
                n303 = call "GExplorer_Queue_GEA2.vi"("Output String"=w1206, "error in (no error)"=w1207) -> ("error out"=w1203:errorcluster)  [unwired: 13 in]
                n304 = call "GEA2 Write ERD.vi"("GEA2 Reference In"=w1199, "GEA Inputs"=w1195, "Write ERD List"=w1200, "Error In"=w1203, "Verify ERD Response?"=FALSE) -> ("GEA2 Reference Out"=w1197:refnum<k24>, "Error Out"=w1196:errorcluster)  [unwired: 8 in, 1 out]
              }
            }
          }
          event "Set Wifi State(ERD 6003)": Value Change {
            n305 = event-data() -> ()  [unwired: 1 in, 6 out]
            n306 = case shown="\"255 - Invalid\"" "Wifi State" {
              tunnel: ["00" "01" "02" "03" "04" "05" "06" "FF"] -> w1237
              frame "0 - OFF", Default {
              }
              frame "1 - App Mode" {
              }
              frame "2 - Connecting" {
              }
              frame "3 - Connected" {
              }
              frame "4 - Connected Off" {
              }
              frame "5 - Scanning" {
              }
              frame "6 - Reconnecting" {
              }
              frame "255 - Invalid" {
              }
            }
            n307 = case shown="True" "Set Wifi State(ERD 6003)" {
              tunnel: w1233 -> [w1238 w1243]
              tunnel: w1234 -> [w1239 w1247]
              tunnel: [w1239 w1245] -> w1232
              tunnel: [w1238 w1246] -> w1231
              tunnel: w1237 -> [_ w1244]
              frame False {
              }
              frame True {
                w1240 = T9 {"Source"=228, "Destination"=191} ("GEA Inputs")
                n308 = Concatenate Strings(w1244) -> (w1256:string)
                n309 = Bundle By Name(cluster=T5 {"ERD Number"=24579, "Data Type"=enum."string", "Data"=""} ("ERD Write Data In"), "Data"=w1256) -> (w1255:T5)
                n310 = Build Array(w1255) -> (w1241:T5[])
                n311 = call "Convert Write ERD List to Message.vi"("GEA Inputs"=w1240, "Write ERD List"=w1241, "Error In"=w1247) -> ("GEA Message"=w1251:T13, "Error Out"=w1252:errorcluster)  [unwired: 11 in]
                n312 = call "GEA2MessageFormatter.vi"("Prefix(Send/Recv)"="SEND", "GEA2 Data In"=w1251, "Error In"=w1252) -> ("Output String"=w1253:string, "Error Out"=w1254:errorcluster)  [unwired: 11 in]
                n313 = call "GExplorer_Queue_GEA2.vi"("Output String"=w1253, "error in (no error)"=w1254) -> ("error out"=w1250:errorcluster)  [unwired: 13 in]
                n314 = call "GEA2 Write ERD.vi"("GEA2 Reference In"=w1243, "GEA Inputs"=w1240, "Write ERD List"=w1241, "Error In"=w1250, "Verify ERD Response?"=FALSE) -> ("GEA2 Reference Out"=w1246:refnum<k24>, "Error Out"=w1245:errorcluster)  [unwired: 8 in, 1 out]
              }
            }
          }
        }
        n315 = call "Error_Control.vi"("Error In"=w683) -> ("Error Out"=w685:errorcluster)  [unwired: 14 in]
      }
      n316 = while "GEA2 Receive Message Loop" {
        shift-right: [w1268] -> w136
        shift-left: w63 -> [w1269]
        shift-right: [w1265] -> _
        shift-left: w48 -> [w1270]
        stop <- w1267 stop-if-true
        # "GEA2 Receive Message Loop"
        n317 = event shown="[0] <Data_Recv>: User Event" {
          selector: w1270 -> [w1281 _ w1304 w1312 w1330]
          dyn-events: [w1281 _ w1304 w1313 w1330] -> w1265
          timeout: _ -> [_ _ _ _ _]
          tunnel: w1269 -> [w1278 w1293 w1296 w1327 w1332]
          tunnel: [w1274 w1293 w1295 w1314 w1332] -> w1266
          tunnel: [FALSE TRUE FALSE _ TRUE] -> w1267
          event User Event {
            w1284 = T13 {"Source"=0, "Destination"=0, "Command"=0, "Message"=""}  # GEA2 Data In
            # "Added subscription Ack"
            n318 = event-data() -> ("Source"=w1283:u8, "Destination"=w1280:u8, "Command"=w1279:u8, "Message"=w1272:string)  [unwired: 1 in]
            n319 = Bundle By Name(cluster=w1284, "Source"=w1283, "Destination"=w1280, "Command"=w1279, "Message"=w1272) -> (w1273:T13)
            n320 = call "GEA2 Log Filter.vi"("Filter Data"="Filter Data", "GEA2 Msg"=w1273, "Cmd to ignore"="Ignore this CMD", "error in (no error)"=w1278) -> ("error out"=w1275:errorcluster)  [unwired: 11 in]
            n321 = property on="Program Ind" class="Bool (strict)"() -> ("Value"=w1271:bool)  [unwired: 2 in, 2 out]
            n322 = case shown="False" w1271 {
              tunnel: w1275 -> [w1290 w1291]
              tunnel: [w1288 w1291] -> w1274
              tunnel: w1273 -> [w1286 _]
              frame False {
                n323 = call "FGV_GEA2_Ref.vi"("Action"=enum16{"Set Ref", "Get Ref"}."Get Ref", "Error In"=w1290) -> ("GEA2 Reference Out"=w1287:refnum<k24>, "Error Out"=w1289:errorcluster)  [unwired: 12 in]
                n324 = call "ACK Subscriptions Publications.vi"("GEA2 Reference In"=w1287, "GEA2 Msg"=w1286, "error in (no error)"=w1289) -> ("error out"=w1288:errorcluster)  [unwired: 11 in, 1 out]
              }
              frame True {
              }
            }
          }
          event User Event {
            n325 = event-data() -> ()  [unwired: 1 in, 7 out]
          }
          event User Event {
            # "This will update the UI with all data sent across the bus via a button Press"
            n326 = event-data() -> ("Source"=w1306:T47, "Destination"=w1303:u8, "Command"=w1302:u8, "Message"=w1301:string)  [unwired: 1 in]
            n327 = Bundle By Name(cluster=T13 {"Source"=0, "Destination"=0, "Command"=0, "Message"=""} ("GEA2 Data In"), "Source"=w1306, "Destination"=w1303, "Command"=w1302, "Message"=w1301) -> (w1297:T13)
            n328 = property on="Program Ind" class="Bool (strict)"() -> ("Value"=w1294:bool)  [unwired: 2 in, 2 out]
            n329 = call "GEA2MessageFormatter.vi"("Prefix(Send/Recv)"="SEND", "GEA2 Data In"=w1297, "Error In"=w1296) -> ("Output String"=w1300:string, "Error Out"=w1298:errorcluster)  [unwired: 11 in]
            n330 = case shown="False" w1294 {
              tunnel: w1300 -> [w1310 _]
              tunnel: w1298 -> [w1309 w1311]
              tunnel: [w1308 w1311] -> w1295
              frame False {
                n331 = call "GExplorer_Queue_GEA2.vi"("Output String"=w1310, "error in (no error)"=w1309) -> ("error out"=w1308:errorcluster)  [unwired: 13 in]
              }
              frame True {
              }
            }
          }
          event "Board Index": Value Change {
            # "Stop old GEA2\nbus reference"
            # "Allow other references a chance\nto begin using new reference"
            # "Store new GEA2 bus reference"
            # "Update event registration\nand initialize new GEA2 bus"
            # "Get the previous GEA2\nbus ref, but don't stop it\nuntil we update the FGV\nwith the new GEA2 ref"
            n332 = event-data() -> ("NewVal"=w1324:u8)  [unwired: 1 in]
            n333 = property on="Board Index" class="DigNum (strict)"(error in=w1327, "DisabledEnum"=T41."Disabled and Grayed Out" ("Disabled")) -> (error out=w1328:errorcluster)  [unwired: 1 in, 1 out]
            n334 = call "FGV_GEA2_Ref.vi"("Action"=enum16{"Set Ref", "Get Ref"}."Get Ref", "Error In"=w1328) -> ("GEA2 Reference Out"=w1318:refnum<k24>, "Error Out"=w1325:errorcluster)  [unwired: 12 in]
            n335 = call "GEA2_Reregister.vi"("Event Registration Refnum"=w1312, "Board Index"=w1324, "Error In"=w1325) -> ("GEA2 Reference Out"=w1323:refnum<k24>, "Event Registration Refnum 2"=w1313:refnum<event-registration>, "Error Out"=w1317:errorcluster)  [unwired: 9 in, 1 out]
            n336 = call "FGV_GEA2_Ref.vi"("GEA2 Reference In"=w1323, "Action"=enum16{"Set Ref", "Get Ref"}."Set Ref", "Error In"=w1317) -> ("Error Out"=w1320:errorcluster)  [unwired: 11 in, 1 out]
            n337 = call "Time Delay"("error in (no error)"=w1320, "Delay Time (s)"=5.0) -> ("error out"=w1319:errorcluster)  [unwired: 9 in]
            n338 = call "GEA2 Stop.vi"("GEA2 Reference In"=w1318, "Error In"=w1319) -> ("Error Out"=w1315:errorcluster)  [unwired: 13 in]
            n339 = property on="Board Index" class="DigNum (strict)"(error in=w1315, "DisabledEnum"=T41."Enabled" ("Disabled")) -> (error out=w1314:errorcluster)  [unwired: 1 in, 1 out]
          }
          event "Stop": Value Change {
            n340 = event-data() -> ()  [unwired: 1 in, 6 out]
          }
        }
        n341 = call "Error_Control.vi"("Error In"=w1266) -> ("Error Out"=w1268:errorcluster)  [unwired: 14 in]
      }
      n342 = while "Continuous Send Loop" {
        shift-right: [w149] -> _
        shift-left: Cont_Send_States."Run" ("State") -> [w148]
        tunnel: w83 -> [w150]
        tunnel: [w143] -> _
        shift-right: [w141] -> w86
        shift-left: w63 -> [w152]
        stop <- w151 stop-if-true
        # "Continuous Send Loop"
        n343 = Dequeue Element(queue=w150, timeout in ms (-1)=0, error in (no error)=w152) -> (queue out=w144:refnum<queue>, element=w137:T36, timed out?=w145:bool, error out=w140:errorcluster)
        n344 = Select(t=w148, s=w145, f=w137) -> (s? t:f=w147:T36)
        n345 = property on="GEA2 Send" class="Clust (strict)"() -> ("Value"=w139:T13)  [unwired: 2 in, 2 out]
        n346 = case shown="\"Run\", Default" w147 {
          selector: w147 -> [w156 w167]
          tunnel: w140 -> [w158 w169]
          tunnel: [w157 w169] -> w142
          tunnel: [_ TRUE] -> w151
          tunnel: [w156 w167] -> w149
          tunnel: w144 -> [w155 w166]
          tunnel: [w155 w166] -> w143
          tunnel: w139 -> [w154 _]
          frame "Run", Default {
            n347 = case shown="True" "Start Send" {
              tunnel: w158 -> [w159 w162]
              tunnel: [w159 w165] -> w157
              tunnel: w154 -> [_ w164]
              frame False {
              }
              frame True {
                n348 = call "FGV_GEA2_Ref.vi"("Action"=enum16{"Set Ref", "Get Ref"}."Get Ref", "Error In"=w162) -> ("GEA2 Reference Out"=w161:refnum<k24>, "Error Out"=w160:errorcluster)  [unwired: 12 in]
                n349 = call "GEA2 Send Message.vi"("GEA2 Reference In"=w161, "Input Data"=w164, "Error In"=w160) -> ("Error Out"=w165:errorcluster)  [unwired: 11 in, 1 out]
              }
            }
          }
          frame "Shutdown" {
          }
        }
        n350 = call "Error_Control.vi"("Error In"=w142) -> ("Error Out"=w141:errorcluster)  [unwired: 14 in]
        n351 = Wait (ms)(milliseconds to wait="Msg Rate (ms)") -> ()  [unwired: 1 out]
      }
      n352 = while "GEA2 Display Loop" {
        tunnel: w64 -> [w400]
        shift-right: [w397] -> _
        shift-left: "" -> [w403]
        shift-right: [w399] -> w120
        shift-left: w80 -> [w407]
        tunnel: w78 -> [w393]
        tunnel: [w391] -> w76
        stop <- w401 stop-if-true
        # "Mensajes de los comandos enviados"
        # "GEA2 Display Loop"
        n353 = Dequeue Element(queue=w400, error in (no error)=w407) -> (element=w406:T40, error out=w402:errorcluster)  [unwired: 1 in, 2 out]
        n354 = Unbundle By Name(w406) -> ("Data"=w404:variant, "State"=w405:enum16{"Add to Log", "Clear", "Shutdown"})
        n355 = case shown="\"Add to Log\", Default" w405 {
          tunnel: w404 -> [w418 _ _]
          tunnel: w403 -> [w421 w426 _]
          tunnel: [w420 w426 ""] -> w398
          tunnel: w402 -> [w419 w427 w431]
          tunnel: [w416 w427 w431] -> w394
          tunnel: [FALSE TRUE FALSE] -> w401
          tunnel: [w408 _ _] -> w392
          frame "Add to Log", Default {
            n356 = Variant To Data(error in=w419, type="", Variant=w418) -> (data=w410:string, error out=w416:errorcluster)
            n357 = String Subset(string=w410, offset (0)=22, length (rest)=7 ("length (rest)")) -> (substring=w411:string)
            n358 = Equal?(x="SEND E5", y=w411) -> (x = y?=w409:bool)
            n359 = case shown="False" w409 {
              tunnel: w421 -> [w424 w425]
              tunnel: [w423 w425] -> w420
              tunnel: w410 -> [w422 _]
              tunnel: [w422 _] -> w408
              frame False {
                n360 = Concatenate Strings(w422, w424) -> (w423:string)
              }
              frame True {
              }
            }
          }
          frame "Shutdown" {
          }
          frame "Clear" {
          }
        }
        "GEA2 Log" <- w398
        n361 = call "Write _To_TXT_File.vi"("refnum"=w393, "text"=w392, "error in"=w394) -> ("refnum out"=w391:refnum<file>, "error out"=w395:errorcluster)  [unwired: 10 in, 1 out]
        n362 = String Subset(string=w398, length (rest)="GEA2 Log Length") -> (substring=w397:string)  [unwired: 1 in]
        n363 = call "Error_Control.vi"("Error In"=w395) -> ("Error Out"=w399:errorcluster)  [unwired: 14 in]
      }
      n364 = while "DAQ Loop" {
        shift-right: [w466] -> w119
        shift-left: w63 -> [w464]
        shift-right: [w450] -> _
        shift-left: DAQ_States."Wait for Init" ("States") -> [w461]
        shift-right: [w451] -> _
        shift-left: "Wait for Init" ("Report Text") -> [w460]
        shift-right: [w449] -> _
        shift-left: _ -> [w442]
        shift-right: [w448] -> _
        shift-left: w67 -> [w447]
        shift-right: [w446] -> _
        shift-left: w67 -> [w445]
        shift-right: [w444] -> _
        shift-left: w67 -> [w443]
        tunnel: w66 -> [w434]
        i -> [w432]
        stop <- w457 stop-if-true
        # "NI 9401 \nMódulo Digital Bidireccionales"
        # "NI 9263 \nMódulo de Salida de Voltaje"
        # "NI 9481 \nModulo de cuatro relevadores"
        # "DAQ Loop"
        n365 = Dequeue Element(queue=w434, timeout in ms (-1)=0, error in (no error)=w464) -> (element=w462:T37, timed out?=w463:bool, error out=w441:errorcluster)  [unwired: 1 out]
        n366 = Wait (ms)(milliseconds to wait=u32 100) -> ()  [unwired: 1 out]
        n367 = Select(t=w461, s=w463, f=w462) -> (s? t:f=w459:T37)
        n368 = case shown="\"Exit\"" w459 {
          selector: w459 -> [_ _ _ _ _ _ w654]
          tunnel: [w471 w481 w498 w534 w588 w604 w639] -> w455
          tunnel: w443 -> [w480 w491 w506 _ w582 w624 w647]
          tunnel: [w480 w491 w506 w526 w580 _ _] -> w444
          tunnel: w445 -> [w479 w489 w507 _ w564 w612 w630]
          tunnel: [w479 w489 w507 w519 w563 _ _] -> w446
          tunnel: [w469 w490 w494 w520 w565 w614 w632] -> w453
          tunnel: [w470 w492 w495 w527 w586 w623 w646] -> w454
          tunnel: [w476 DAQ_States."Verify Hardware" ("States") w503 DAQ_States."Run" ("States") w589 DAQ_States."Wait for Init" ("States") w654] -> w450
          tunnel: [FALSE FALSE FALSE TRUE TRUE FALSE FALSE] -> w449
          tunnel: [_ _ _ _ _ FALSE TRUE] -> w457
          tunnel: [w468 w488 w493 w514 w561 w602 w652] -> w452
          tunnel: [w478 w487 w508 w513 w559 _ _] -> w448
          tunnel: w447 -> [w478 w487 w508 _ w560 w601 w653]
          tunnel: [w477 "Rename Devices" ("Report Text") w500 "Initialize" ("Report Text") "Running" ("Report Text") "Wait for Init" ("Report Text") "Exit" ("Report Text")] -> w451
          tunnel: w460 -> [w477 _ _ _ _ _ _]
          tunnel: "Turn On DAQ" -> [w472 _ _ _ w587 _ _]
          tunnel: w441 -> [w471 w482 w496 w534 w588 w621 w640]
          tunnel: w441 -> [w470 w492 w495 w528 w576 w625 w648]
          tunnel: w441 -> [w469 w490 w494 w521 w566 w613 w631]
          tunnel: w441 -> [w468 w488 w493 w518 w562 w603 w650]
          tunnel: w442 -> [_ _ _ _ _ _ w649]
          tunnel: [_ _ _ _ w557 _ _] -> w440
          tunnel: [_ _ _ _ w556 _ _] -> w439
          tunnel: [_ _ _ _ w554 _ _] -> w438
          tunnel: [_ _ _ _ w553 _ _] -> w437
          tunnel: [_ _ _ _ w552 _ _] -> w436
          tunnel: [_ _ _ _ w549 _ _] -> w435
          tunnel: [_ _ _ _ w548 _ _] -> w433
          tunnel: w432 -> [_ _ _ _ w547 _ _]
          frame "Wait for Init", Default {
            # "DIO"
            # "Relays"
            # "AO"
            n369 = Select(t=DAQ_States."Rename Devices", s=w472, f=DAQ_States."Wait for Init" ("States")) -> (s? t:f=w476:T37)
          }
          frame "Rename Devices" {
            # "DIO"
            # "Relays"
            # "AO"
            n370 = call "Rename DAQ Devices.vi"("cDAQ Name"="JL_SLB", "Error In"=w482) -> ("Error Out"=w481:errorcluster)  [unwired: 13 in]
          }
          frame "Verify Hardware" {
            # "DIO"
            # "Relays"
            # "AO"
            n371 = call "DeviceListCheck.vi"("Device List"=string[] ["9401_1", "9481_1", "9263_1"], "Error In"=w496) -> ("Devices Present?"=w497:bool, "Report Text"=w500:string, "Error Out"=w499:errorcluster)  [unwired: 11 in]
            n372 = case shown="False" w497 {
              selector: w497 -> [w510 _]
              tunnel: w499 -> [w511 w512]
              tunnel: [w509 w512] -> w498
              frame False {
                n373 = property on="Turn On DAQ" class="Bool (strict)"(error in=w511, "Value"=w510) -> (error out=w509:errorcluster)  [unwired: 1 in, 1 out]
              }
              frame True {
              }
            }
            n374 = Select(t=DAQ_States."Initialize" ("f"), s=w497, f=DAQ_States."Wait for Init") -> (s? t:f=w503:T37)
          }
          frame "Initialize" {
            w516 = 0 items=["one channel for each line", "one channel for all lines"] ("line grouping")
            w523 = 0.0  # minimum value
            w524 = 5.0  # maximum value
            w531 = 0 items=["one channel for each line", "one channel for all lines"] ("line grouping")
            # "DIO"
            # "Relays"
            # "AO"
            n375 = call-poly <vilib>:"DAQmx Create Virtual Channel.vi"("lines"=tag "9481_1/port0/line0:3", "name to assign"="Relays", "line grouping"=w531, "error in"=w528) -> ("task out"=w526:refnum<k21>, "error out"=w527:errorcluster)  [unwired: 10 in]
            n376 = call-poly <vilib>:"DAQmx Create Virtual Channel.vi"("maximum value"=w524, "minimum value"=w523, "physical channels"=tag "9263_1/ao0:2" ("lines"), "name to assign"="AO", "error in"=w521) -> ("task out"=w519:refnum<k21>, "error out"=w520:errorcluster)  [unwired: 9 in]
            n377 = call-poly <vilib>:"DAQmx Create Virtual Channel.vi"("lines"=tag "9401_1/port0/line0:5", "name to assign"="DIO", "line grouping"=w516, "error in"=w518) -> ("task out"=w513:refnum<k21>, "error out"=w514:errorcluster)  [unwired: 10 in]
          }
          frame "Run" {
            # "DIO"
            # "Relays"
            # "AO"
            n378 = call-poly <vilib>:"DAQmx Read.vi"("task/channels in"=w560, "error in"=w562) -> ("task out"=w559:refnum<k21>, "data"=w558:bool[], "error out"=w561:errorcluster)  [unwired: 11 in]
            n379 = property on="Drum" class="Bool (strict)"() -> ("Value"=w550:bool)  [unwired: 2 in, 2 out]
            n380 = call "Outlet Convert Temp to Volt.vi"("Model IN"="Model", "Outlet Temperature"="Outlet Therm (F)", "Error In"=w566) -> ("Outlet Voltage"=w538:dbl, "Error Out"=w573:errorcluster)  [unwired: 11 in]
            "Outlet Voltage" <- w538
            n381 = Select(t=w550, s="CentSWControlType", f="CentSWControl") -> (s? t:f=w549:bool)
            n382 = Not(x="Normal Temp V") -> (.not. x?=w539:bool)
            n383 = Index Array(array=w558) -> (element #1=w557:bool, element #2=w556:bool, element #3=w555:bool, element #4=w553:bool, element #5=w552:bool, element #6=w548:bool)  [unwired: 6 in]
            n384 = case shown="True" "CentSWControlType" {
              tunnel: [T41."Enabled" ("Disabled") T41."Disabled and Grayed Out" ("Disabled")] -> w579
              tunnel: [w596 w598] -> w577
              tunnel: w576 -> [w596 w598]
              frame False {
              }
              frame True {
              }
            }
            n385 = call "Inlet_Temp_To_Voltage.vi"("Model"=enum16{"Estar Centauro", "GFL"}."GFL", "Temperature"="Inlet Therm (F)", "Error In"=w573) -> ("Voltage"=w541:dbl, "Error Out"=w572:errorcluster)  [unwired: 11 in]
            "Inlet Voltage" <- w541
            n386 = case shown="True" w555 {
              tunnel: ["CCW" "CW"] -> w554
              frame False {
              }
              frame True {
              }
            }
            n387 = Select(t="Manual Inlet", s=w539, f=w541) -> (s? t:f=w542:dbl)
            n388 = property on="CentSWControl" class="Bool (strict)"(error in=w577, "DisabledEnum"=w579) -> (error out=w578:errorcluster)  [unwired: 1 in, 1 out]
            n389 = Select(t="Manual Outlet", s=w539, f=w538) -> (s? t:f=w544:dbl)
            n390 = call "Dither.vi"("Moisture (V) in"="Moisture (V)", "Dither"="Dither (V)", "Iteration Terminal"=w547, "Error In"=w572) -> ("Moisture (V)"=w568:dbl, "Error Out"=w571:errorcluster)  [unwired: 10 in]
            n391 = Select(t=DAQ_States."Run" ("States"), s=w587, f=DAQ_States."Shutdown" ("States")) -> (s? t:f=w589:T37)
            n392 = Build Array(w549, "Door Status", "AC Power", "Start Signal") -> (w581:bool[])
            n393 = Build Array(w544, w542, w568) -> (w574:dbl[])
            n394 = call-poly <vilib>:"DAQmx Write.vi"("task/channels in"=w582, "data"=w581, "error in"=w578) -> ("task out"=w580:refnum<k21>, "error out"=w586:errorcluster)  [unwired: 10 in, 1 out]
            n395 = call-poly <vilib>:"DAQmx Write.vi"("task/channels in"=w564, "data"=w574, "error in"=w571) -> ("task out"=w563:refnum<k21>, "error out"=w565:errorcluster)  [unwired: 10 in, 1 out]
          }
          frame "Shutdown" {
            w619 = 0.0
            # "This Value is Gets You within 20 \nof Thershold of 2400         ===>"
            # "DIO"
            # "Relays"
            # "AO"
            n396 = property on="Turn On DAQ" class="Bool (strict)"(error in=w621, "Value"=FALSE ("Turn On DAQ")) -> (error out=w607:errorcluster)  [unwired: 1 in, 1 out]
            n397 = property on="CentSWControlType" class="Bool (strict)"(error in=w607, "Value"=TRUE ("CentSWControlType")) -> (error out=w605:errorcluster)  [unwired: 1 in, 1 out]
            n398 = Build Array(w619, w619, w619) -> (w620:dbl[])
            n399 = call-poly <vilib>:"DAQmx Write.vi"("task/channels in"=w612, "data"=w620, "error in"=w613) -> ("task out"=w600:refnum<k21>, "error out"=w618:errorcluster)  [unwired: 10 in, 1 out]
            n400 = call <vilib>:"DAQmx Clear Task.vi"("task in"=w601, "error in"=w603) -> ("error out"=w602:errorcluster)  [unwired: 13 in]
            n401 = call <vilib>:"DAQmx Clear Task.vi"("task in"=w624, "error in"=w625) -> ("error out"=w623:errorcluster)  [unwired: 13 in]
            n402 = call <vilib>:"DAQmx Clear Task.vi"("task in"=w600, "error in"=w618) -> ("error out"=w617:errorcluster)  [unwired: 13 in]
            n403 = property on="Outlet Therm (F)" class="Knob (strict)"(error in=w617, "Value"=75.0 ("Outlet Therm (F)")) -> (error out=w616:errorcluster)  [unwired: 1 in, 1 out]
            n404 = property on="CentSWControl" class="Bool (strict)"(error in=w605, "DisabledEnum"=T41."Disabled and Grayed Out" ("Disabled")) -> (error out=w604:errorcluster)  [unwired: 1 in, 1 out]
            n405 = property on="Inlet Therm (F)" class="Knob (strict)"(error in=w616, "Value"=75.0 ("Inlet Therm (F)")) -> (error out=w615:errorcluster)  [unwired: 1 in, 1 out]
            n406 = property on="Moisture (V)" class="Slide (strict)"(error in=w615, "Value"=1.84511 ("Moisture (V)")) -> (error out=w614:errorcluster)  [unwired: 1 in, 1 out]
          }
          frame "Exit" {
            # "This Value is Gets You within 20 \nof Thershold of 2400         ===>"
            n407 = case shown="True" w649 {
              tunnel: w647 -> [_ w672]
              tunnel: [w657 w671] -> w633
              tunnel: [w659 w670] -> w646
              tunnel: w653 -> [_ w669]
              tunnel: [w658 w668] -> w652
              tunnel: w648 -> [w659 w667]
              tunnel: w650 -> [w658 w666]
              tunnel: w631 -> [w657 w661]
              tunnel: w630 -> [_ w660]
              frame False {
              }
              frame True {
                w664 = 0.0
                # "DIO"
                # "Relays"
                # "AO"
                n408 = Build Array(w664, w664, w664) -> (w665:dbl[])
                n409 = call-poly <vilib>:"DAQmx Write.vi"("task/channels in"=w660, "data"=w665, "error in"=w661) -> ("task out"=w663:refnum<k21>, "error out"=w662:errorcluster)  [unwired: 10 in, 1 out]
                n410 = call <vilib>:"DAQmx Clear Task.vi"("task in"=w672, "error in"=w667) -> ("error out"=w670:errorcluster)  [unwired: 13 in]
                n411 = call <vilib>:"DAQmx Clear Task.vi"("task in"=w663, "error in"=w662) -> ("error out"=w671:errorcluster)  [unwired: 13 in]
                n412 = call <vilib>:"DAQmx Clear Task.vi"("task in"=w669, "error in"=w666) -> ("error out"=w668:errorcluster)  [unwired: 13 in]
              }
            }
            n413 = property on="Turn On DAQ" class="Bool (strict)"(error in=w640, "Value"=FALSE ("Turn On DAQ")) -> (error out=w643:errorcluster)  [unwired: 1 in, 1 out]
            n414 = property on="CentSWControlType" class="Bool (strict)"(error in=w643, "Value"=TRUE ("CentSWControlType")) -> (error out=w641:errorcluster)  [unwired: 1 in, 1 out]
            n415 = property on="Outlet Therm (F)" class="Knob (strict)"(error in=w633, "Value"=75.0 ("Outlet Therm (F)")) -> (error out=w638:errorcluster)  [unwired: 1 in, 1 out]
            n416 = property on="CentSWControl" class="Bool (strict)"(error in=w641, "DisabledEnum"=T41."Disabled and Grayed Out" ("Disabled")) -> (error out=w639:errorcluster)  [unwired: 1 in, 1 out]
            n417 = property on="Inlet Therm (F)" class="Knob (strict)"(error in=w638, "Value"=75.0 ("Inlet Therm (F)")) -> (error out=w637:errorcluster)  [unwired: 1 in, 1 out]
            n418 = property on="Moisture (V)" class="Slide (strict)"(error in=w637, "Value"=1.84511 ("Moisture (V)")) -> (error out=w632:errorcluster)  [unwired: 1 in, 1 out]
          }
        }
        "DAQ Status" <- w451
        "DAQ On?" <- w449
        "Steam" <- w440
        "Drum" <- w439
        "Drum Direction" <- w438
        "Inner/Gas Coil" <- w437
        "Outer Coil" <- w436
        "Drum Light" <- w433
        "Centrifugal Switch" <- w435
        n419 = Merge Errors(w455, w454, w453, w452) -> (w456:errorcluster)
        n420 = call "Error_Control.vi"("Error In"=w456) -> ("Error Out"=w466:errorcluster)  [unwired: 14 in]
      }
      n421 = Close File(refnum=w76, error in=w120) -> (error out=w77:errorcluster)  [unwired: 1 out]
      n422 = call "GEA2 Stop.vi"("GEA2 Reference In"=w134, "Error In"=w135) -> ("Error Out"=w129:errorcluster)  [unwired: 13 in]
      n423 = Close File(refnum=w90, error in=w92) -> (error out=w91:errorcluster)  [unwired: 1 out]
      n424 = Merge Errors(w91, w77, w86, w136, w129, w119) -> (w117:errorcluster)
      n425 = Obtain Queue(name (unnamed)="Continuous Send", element data type=Cont_Send_States."Run" ("State")) -> (queue out=w89:refnum<queue>, error out=w88:errorcluster)  [unwired: 3 in, 1 out]
      n426 = Obtain Queue(name (unnamed)="ERD Loop", element data type=T38 {"Data"=variant, "State"=enum."Read ERDs"} ("Data"), error in (no error)=w117) -> (queue out=w126:refnum<queue>, error out=w125:errorcluster)  [unwired: 2 in, 1 out]
      n427 = Obtain Queue(name (unnamed)="GEA2", element data type=T40 {"Data"=variant, "State"=enum."Add to Log"} ("Data"), error in (no error)=w117) -> (queue out=w133:refnum<queue>, error out=w132:errorcluster)  [unwired: 2 in, 1 out]
      n428 = Obtain Queue(name (unnamed)="DAQ", element data type=DAQ_States."Wait for Init" ("States"), error in (no error)=w117) -> (queue out=w121:refnum<queue>, error out=w122:errorcluster)  [unwired: 2 in, 1 out]
      n429 = Release Queue(queue=w89, error in (no error)=w88) -> (error out=w87:errorcluster)  [unwired: 1 in, 2 out]
      n430 = Release Queue(queue=w126, error in (no error)=w125) -> (error out=w114:errorcluster)  [unwired: 1 in, 2 out]
      n431 = Release Queue(queue=w133, error in (no error)=w132) -> (error out=w115:errorcluster)  [unwired: 1 in, 2 out]
      n432 = Release Queue(queue=w121, error in (no error)=w122) -> (error out=w116:errorcluster)  [unwired: 1 in, 2 out]
      n433 = Merge Errors(w87, w114, w115, w116) -> (w113:errorcluster)
      n434 = call "Error_Control.vi"("Command (Handle Errors)"=Error_Command."Report Errors", "Error In"=w113) -> ("Error Out"=w112:errorcluster)  [unwired: 13 in]
    }
    frame Error {
    }
  }
  n435 = call <vilib>:"Simple Error Handler.vi"("error in (no error)"=w27) -> ("error out"=→"Error Out":errorcluster)  [unwired: 4 in, 4 out]
